vi "ReversedEngineering GetClassDependencyInfo.vi"(1 "Class/Create Path":path=path "C:/classes/P1S/EG1_class/EG1.lvclass", 5 "error in (no error)":errorcluster, 7 "Only analyse this class methods and attributes(False)":bool) -> (15 "classInfo":T5, 16 "TypeDefs":T1[](array[typedef]), 19 "error out":errorcluster)   [LabVIEW 2020]
doc: "Gets current diagram values"
uses:
  <resource>/Framework/Providers/Open_GDS/UML/ReversedEngineering/ReversedEngineering ClassInfoType.ctl
  <resource>/Framework/Providers/Open_GDS/UML/UMLEditor/UMLEditor_VisibilityType.ctl
  <resource>/Framework/Providers/Open_GDS/UML/ReversedEngineering/ReversedEngineering AttributeInfoType.ctl
  <resource>/Framework/Providers/Open_GDS/ClassProviders/Common/CommonVIs/CommonVIs_AttributeDataType.ctl
  <resource>/Framework/Providers/Open_GDS/UML/ReversedEngineering/ReversedEngineering_ClassDependencyDetailsType.ctl
  <resource>/Framework/Providers/Open_GDS/ClassProviders/Common/ScriptingFunctions/SubVIs/Scripting_ViDependencyType.ctl
  <resource>/Framework/Providers/Open_GDS/UML/ReversedEngineering/ReversedEngineering TypeDefType.ctl
  <resource>/Framework/Providers/Open_GDS/ClassProviders/Provider_BaseClassInterface/ClassReader_class/MethodDependencyType.ctl
  <resource>/Framework/Providers/Open_GDS/UML/UMLEditor/UMLEditor BusyDialogAction.ctl
  <resource>/Framework/Providers/Open_GDS/ClassProviders/Provider_BaseClassInterface/ClassReader_class/ClassReader.lvclass
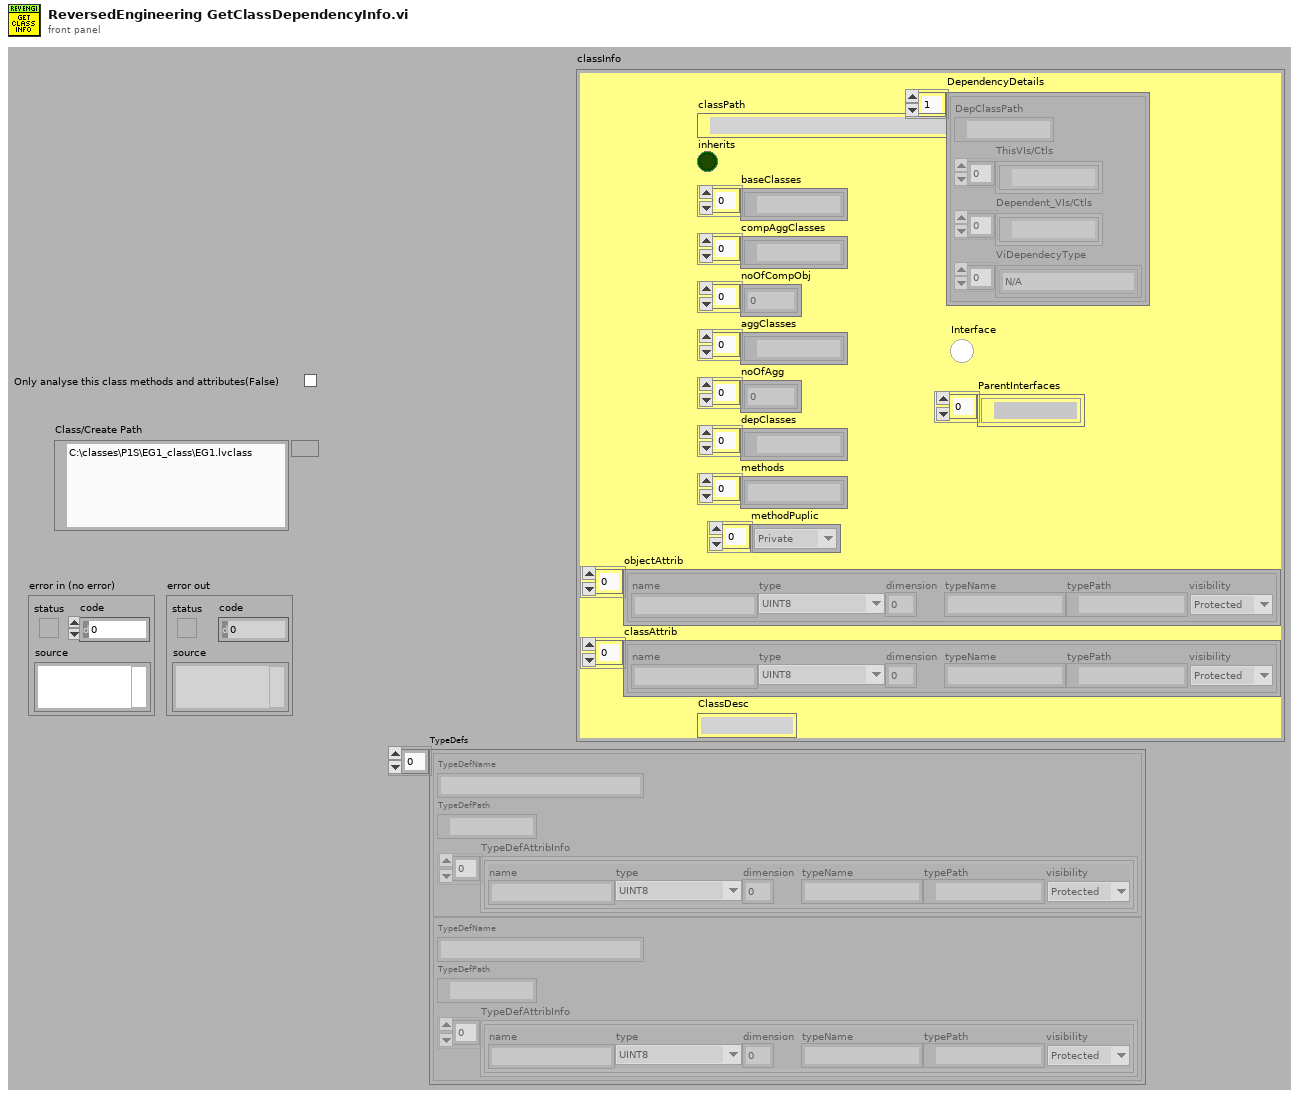
[diagram p1: front panel]
types:
  T1 = typedef "ReversedEngineering TypeDefType.ctl" = cluster{"TypeDefName":string, "TypeDefPath":path, "TypeDefAttribInfo":T2[]}
  T2 = typedef "ReversedEngineering AttributeInfoType.ctl" = cluster{"name":string, "type":T3, "dimension":i32, "typeName":string, "typePath":path, "visibility":T4}
  T3 = typedef "CommonVIs_AttributeDataType.ctl" = enum16{"UINT8", "INT8", "UINT16", "INT16", "UINT32", "INT32", "UINT64", "INT64", "SGL", "DBL", "EXT", "CSG", "CDB", "CXT", "TimeStamp", "STRING", "PATH", "BOOL", "ENUM", "RefNum", "VIRefNum", "LabVIEW Class", "Cluster", "Variant", "TypeDef", "Waveform", "LabVIEW Object", "Other", "void", "Set", "Map"}
  T4 = typedef "UMLEditor_VisibilityType.ctl" = enum16{"Public", "Private", "Protected"}
  T5 = typedef "ReversedEngineering ClassInfoType.ctl" = cluster{"classPath":path, "inherits":bool, "baseClasses":path[], "compAggClasses":path[], "noOfCompObj":i32[], "aggClasses":path[], "noOfAgg":i32[], "depClasses":path[], "methods":string[], "methodPuplic":T4[], "objectAttrib":T2[], "classAttrib":T2[], "ClassDesc":string, "DependencyDetails":T6[], "Interface":bool, "ParentInterfaces":path[]}
  T6 = typedef "ReversedEngineering_ClassDependencyDetailsType.ctl" = cluster{"DepClassPath":path, "ThisVIs/Ctls":path[], "Dependent_VIs/Ctls":path[], "ViDependecyType":T7[]}
  T7 = typedef "Scripting_ViDependencyType.ctl" = enum16{"N/A", "Launches"}
  T8 = typedef "MethodDependencyType.ctl" = cluster{"Method/VI":path, "SubVIs/Ctls":path[], "SubVIClassOwner":string[], "ClassMethodName":string[], "SubVIClassOwnerPath":path[], "DepType":T7[]}
  T9 = cluster{"inherits":bool, "baseClasses":path[], "compositeAggregationClassPath":path[], "noOfCompositeObjects":i32[], "aggregationClassPath":path[], "noOfAggObjects":i32[], "dependencyClassPath":path[], "className":string, "classPath":path, "createRef":refnum<vi>, "depClassDescRefs":refnum<vi>[], "createPath":path, "depClassNames":string[], "depClassPaths":path[], "noOfObjects1":i32[], "refData":string, "refType":i16[], "noOfObjects2":i32[], "depTypeDefsVIs":path[], "depTypeDefsClassPath":path[], "depCreateClassPaths":path[], "objectRefsInAttrib":path[], "objectRefClassesInAttrib":path[], "objectRefInAttribIsAnArray":bool[], "methodNames":string[], "objectAttribInfo":T2[], "classAttribInfo":T2[], "errMsg":string, "dirClass":bool, "CreateClassVIsCalled":path[], "TypeDefs":T1[], "ClassDesc":string, "DependencyDetails":T6[], "methodPuplic":T4[], "depMethodVIs":T8[], "DataFlowClass":bool, "IsDependencyClassPathsAByValueClass":bool[], "Interface":bool, "ParentInterfaces":path[]}
  T10 = typedef "UMLEditor BusyDialogAction.ctl" = enum16{"Initialize", "Open(VIs)", "Open(i)", "Send_I-Value", "SendStatusMessage", "GetBusyDialogStatus", "Close", "Quit"}
  T11 = enum16{"NormalSubVis", "LV-Internal VIs", "All VIs", "All Functions"}
  T12 = enum32{"invalid VI type", "Standard VI", "Control VI", "Global VI", "Polymorphic VI", "Configuration VI", "SubSystem", "Facade VI", "Method VI", "Statechart Diagram VI"}
  T13 = enum32{"invalid scope", "public", "private", "protected", "community"}
  T14 = typedef "ClassTypes_MethodType.ctl" = cluster{"MethodName":string, "Visibility":enum16{"Public", "Private", "Protected"}, "StereoType":string, "Path":path}
  T15 = typedef "Librarian File Info Out.ctl" = cluster{"creation date":u32, "last mod date":u32, "type":string, "creator":string, "LV version":i32, "size":i32, "top level":bool}
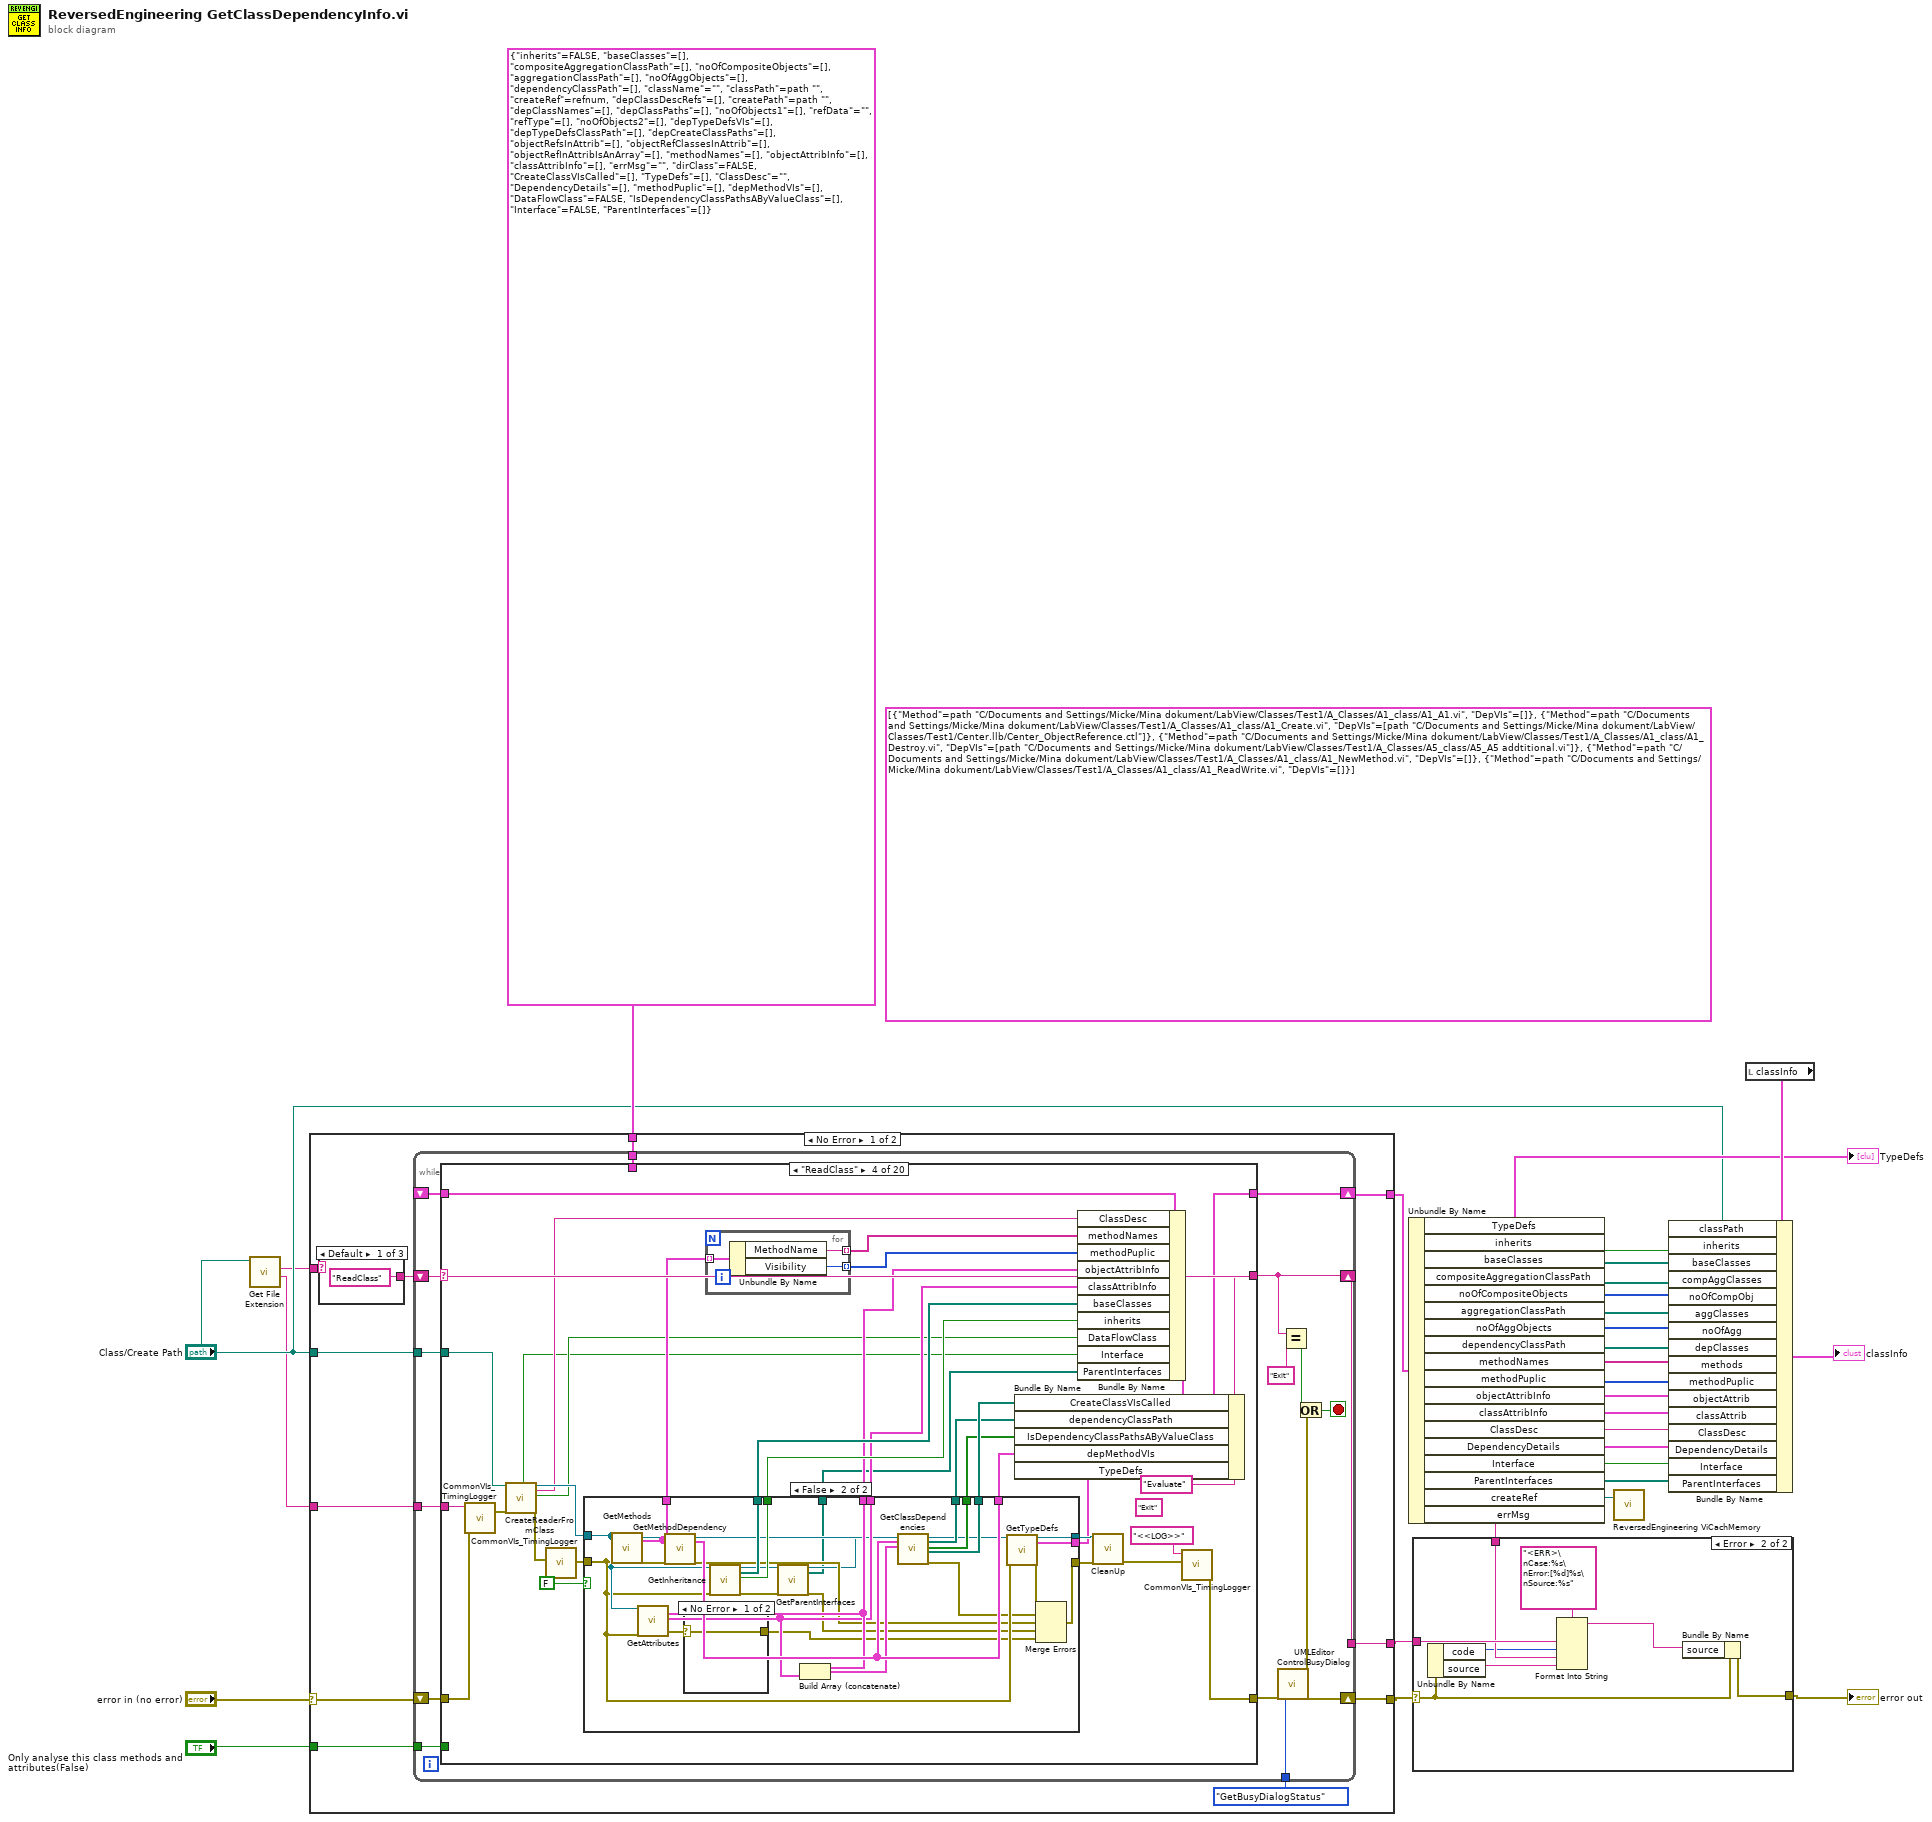
[diagram p0: block diagram]
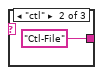
[diagram p3: hidden frame]
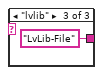
[diagram p4: hidden frame]
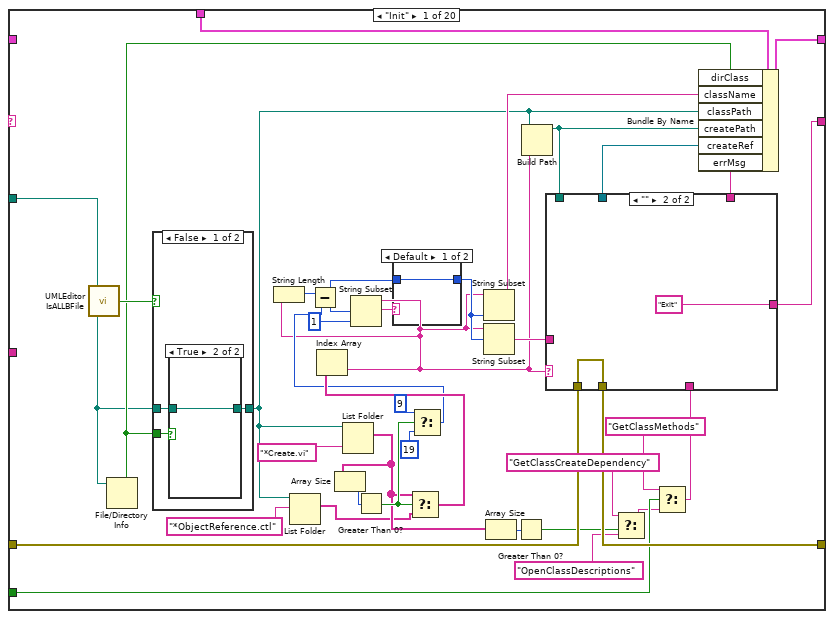
[diagram p5: hidden frame]
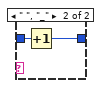
[diagram p6: hidden frame]
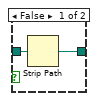
[diagram p7: hidden frame]
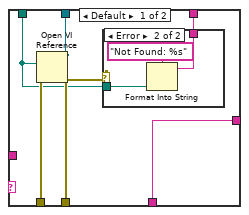
[diagram p9: hidden frame]
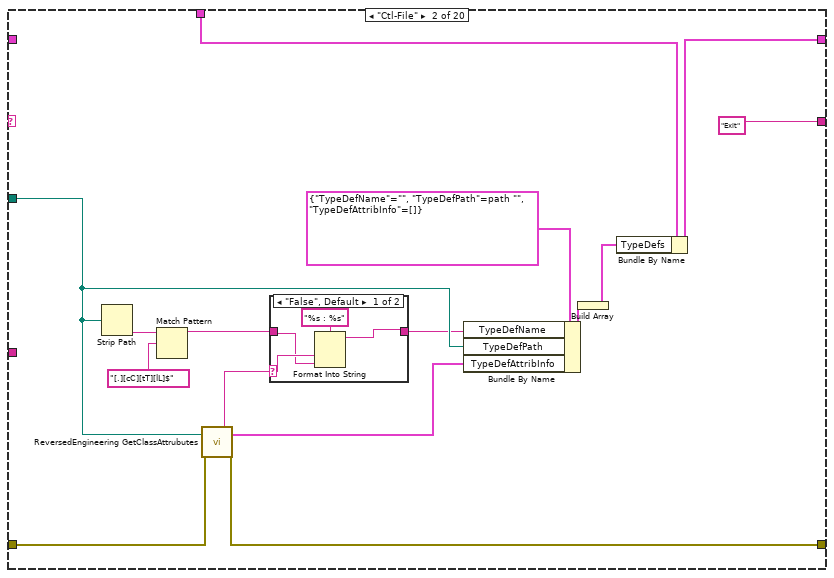
[diagram p11: hidden frame]
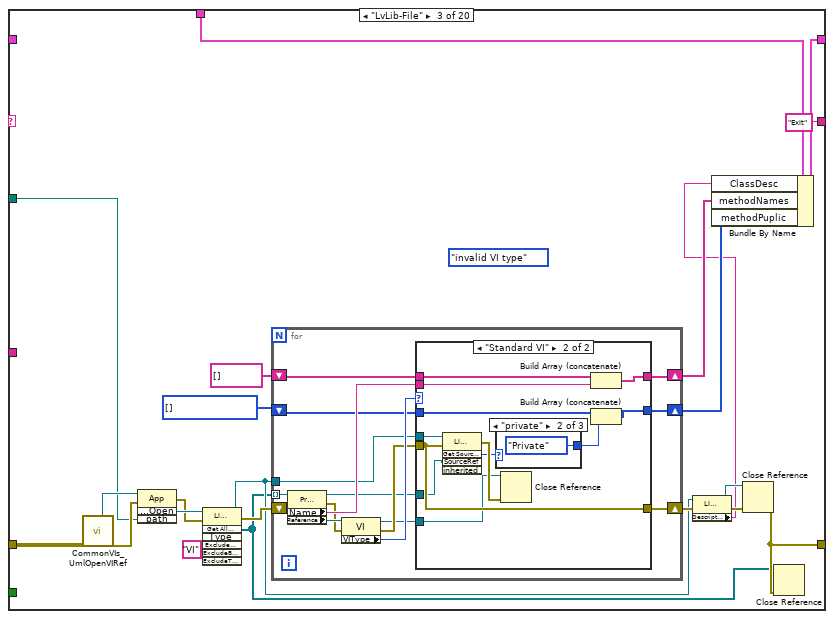
[diagram p13: hidden frame]
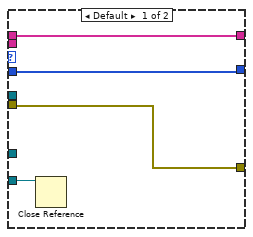
[diagram p14: hidden frame]
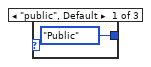
[diagram p15: hidden frame]
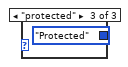
[diagram p16: hidden frame]
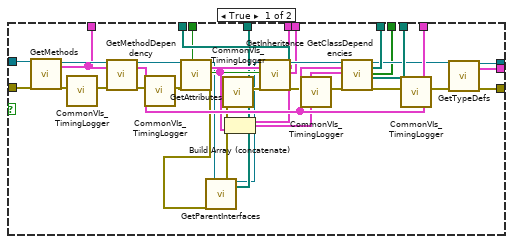
[diagram p17: hidden frame]
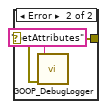
[diagram p18: hidden frame]
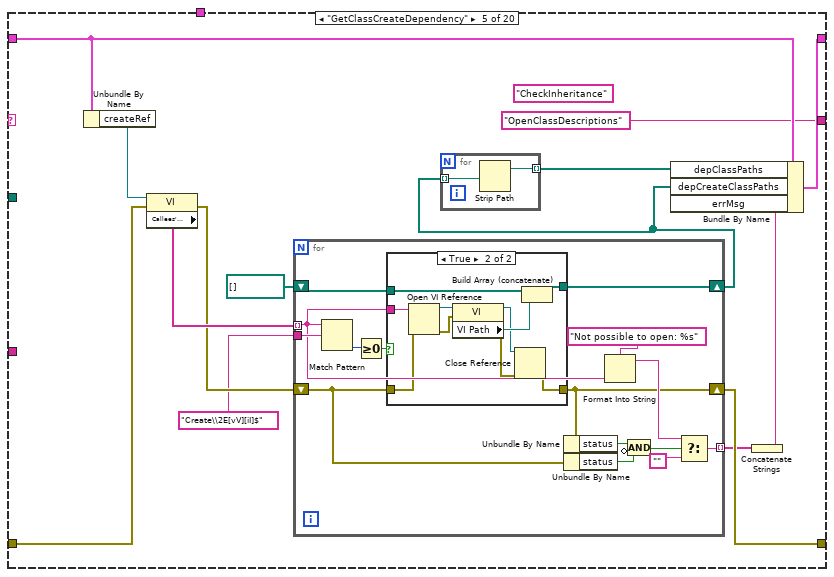
[diagram p19: hidden frame]
diagram:
  (unwired) cluster{"Method":path, "DepVIs":path[]}[] [{"Method"=path "C:/Documents and Settings/Micke/Mina dokument/LabView/Classes/Test1/A_Classes/A1_class/A1_A1.vi", "DepVIs"=[]}, {"Method"=path "C:/Documents and Settings/Micke/Mina dokument/LabView/Classes/Test1/A_Classes/A1_class/A1_Create.vi", "DepVIs"=[path "C:/Documents and Settings/Micke/Mina dokument/LabView/Classes/Test1/Center.llb/Center_ObjectReference.ctl"]}, {"Method"=path "C:/Documents and Settings/Micke/Mina dokument/LabView/Classes/Test1/A_Classes/A1_class/A1_Destroy.vi", "DepVIs"=[path "C:/Documents and Settings/Micke/Mina dokument/LabView/Classes/Test1/A_Classes/A5_class/A5_A5 addtitional.vi"]}, {"Method"=path "C:/Documents and Settings/Micke/Mina dokument/LabView/Classes/Test1/A_Classes/A1_class/A1_NewMethod.vi", "DepVIs"=[]}, {"Method"=path "C:/Documents and Settings/Micke/Mina dokument/LabView/Classes/Test1/A_Classes/A1_class/A1_ReadWrite.vi", "DepVIs"=[]}] ("depMethodVIs")
  n1 = call <vilib>:"Get File Extension.vi"("file"="Class/Create Path") -> ("filename without extension"=w3:string, "lowercase file extension"=w4:string)  [unwired: 1 in, 8 out]
  n2 = case shown="No Error" "error in (no error)" {
    selector: "error in (no error)" -> [w41 w1100]
    tunnel: [w40 w1100] -> w15
    tunnel: "Class/Create Path" -> [w39 _]
    tunnel: [w38 _] -> w29
    tunnel: [w37 _] -> w13
    tunnel: "Only analyse this class methods and attributes(False)" -> [w36 _]
    tunnel: T9 {"inherits"=FALSE, "baseClasses"=[], "compositeAggregationClassPath"=[], "noOfCompositeObjects"=[], "aggregationClassPath"=[], "noOfAggObjects"=[], "dependencyClassPath"=[], "className"="", "classPath"=path "", "createRef"=refnum, "depClassDescRefs"=[], "createPath"=path "", "depClassNames"=[], "depClassPaths"=[], "noOfObjects1"=[], "refData"="", "refType"=[], "noOfObjects2"=[], "depTypeDefsVIs"=[], "depTypeDefsClassPath"=[], "depCreateClassPaths"=[], "objectRefsInAttrib"=[], "objectRefClassesInAttrib"=[], "objectRefInAttribIsAnArray"=[], "methodNames"=[], "objectAttribInfo"=[], "classAttribInfo"=[], "errMsg"="", "dirClass"=FALSE, "CreateClassVIsCalled"=[], "TypeDefs"=[], "ClassDesc"="", "DependencyDetails"=[], "methodPuplic"=[], "depMethodVIs"=[], "DataFlowClass"=FALSE, "IsDependencyClassPathsAByValueClass"=[], "Interface"=FALSE, "ParentInterfaces"=[]} ("Cluster") -> [w34 _]
    tunnel: w4 -> [w33 _]
    tunnel: w3 -> [w31 _]
    frame No Error {
      n3 = case shown="Default" w33 {
        tunnel: ["ReadClass" ("y") "Ctl-File" "LvLib-File"] -> w32
        frame Default {
        }
        frame "ctl" {
        }
        frame "lvlib" {
        }
      }
      n4 = while {
        shift-right: [w58] -> _
        shift-left: w32 -> [w51]
        shift-right: [w45] -> w40
        shift-left: w41 -> [w59]
        shift-right: [w53] -> w38
        shift-left: _ -> [w54]
        tunnel: w39 -> [w52]
        tunnel: [w51] -> w37
        tunnel: w36 -> [w50]
        tunnel: UMLEditor_BusyDialogAction."GetBusyDialogStatus" ("Action(SendStatusMessage)") -> [w48]
        tunnel: w34 -> [w47]
        tunnel: w31 -> [w46]
        stop <- w55 stop-if-true
        n5 = case shown="\"ReadClass\"" w51 {
          tunnel: w59 -> [w87 w133 w156 w202 w306 w340 w368 w433 w479 w575 w661 w681 w703 w726 w791 w813 w879 w954 w1018 w1097]
          tunnel: [w86 w131 w140 w196 w302 w336 w369 w433 w460 w575 w666 w694 w701 w726 w791 w813 w879 w954 w1018 w1097] -> w49
          tunnel: [w96 "Exit" ("y") "Exit" ("y") "Evaluate" ("y") "OpenClassDescriptions" ("y") "CheckInheritance" ("y") "GetMultiplicity" ("y") "GetClassMethods" ("y") "GetClassMethodDepenencies" ("y") "GetObjectAttributsDepenencies" ("y") "GetClassAttributsDepenencies" ("y") "CloseRefs" ("y") "Evaluate" ("y") "RemoveInheritDependency" ("y") "CreateTypeDefs?" ("y") "AddReferencedTypeDefs" ("y") "UpdateTypeDefsAttribName?" ("y") "SortMethodToClassDependencies" ("y") "Exit" ("y") "Exit" ("y")] -> w58
          tunnel: w54 -> [_ _ _ w225 w301 w358 w365 w436 w474 w571 w668 w689 w702 w710 w789 w808 w881 w961 w1017 w1099]
          tunnel: [w95 w130 w158 w216 w300 w359 w373 w438 w475 w576 w669 w690 w702 w725 w790 w815 w880 w960 w1019 w1099] -> w53
          tunnel: w52 -> [w68 w126 w155 w226 _ _ _ _ _ _ _ _ _ _ _ _ _ _ _ _]
          tunnel: w50 -> [w71 _ _ _ _ _ _ _ _ _ _ _ _ _ _ _ _ _ _ _]
          tunnel: w47 -> [w60 w122 w141 _ _ _ _ _ _ _ _ _ _ _ _ _ _ _ _ _]
          tunnel: w46 -> [_ _ _ w201 _ _ _ _ _ _ _ _ _ _ _ _ _ _ _ _]
          frame "Init" {
            n6 = call <resource>:"UMLEditor IsALLBFile.vi"("path"=w68) -> ("path to VI library?"=w97:bool)
            n7 = File/Directory Info(path=w68) -> (directory=w84:bool)  [unwired: 1 in, 6 out]
            n8 = case shown="False" w97 {
              tunnel: w68 -> [w103 w107]
              tunnel: [w102 w107] -> w64
              tunnel: w84 -> [w101 _]
              frame False {
                n9 = case shown="True" w101 {
                  tunnel: w103 -> [w105 w106]
                  tunnel: [w104 w106] -> w102
                  frame False {
                    n10 = Strip Path(path=w105) -> (stripped path=w104:path)  [unwired: 1 out]
                  }
                  frame True {
                  }
                }
              }
              frame True {
              }
            }
            n11 = List Folder(path=w64, pattern="*ObjectReference.ctl") -> (filenames=w62:string[])  [unwired: 1 in, 4 out]
            n12 = List Folder(path=w64, pattern="*Create.vi") -> (filenames=w67:string[])  [unwired: 1 in, 4 out]
            n13 = Array Size(array=w67) -> (size(s)=w81:i32)
            n14 = Greater Than 0?(x=w81) -> (x > 0?=w79:bool)
            n15 = Select(t=w67, s=w79, f=w62) -> (s? t:f=w80:string[])
            n16 = Index Array(array=w80) -> (element=w65:string)  [unwired: 1 in]
            n17 = String Length(string=w65) -> (length=w83:i32)
            n18 = Select(t=9 ("y"), s=w79, f=19 ("y")) -> (s? t:f=w76:i32)
            n19 = Subtract(x=w83, y=w76) -> (x-y=w82:i32)
            n20 = String Subset(string=w65, offset (0)=w82, length (rest)=1 ("length (rest)")) -> (substring=w89:string)
            n21 = case shown="Default" w89 {
              tunnel: w82 -> [w98 w100]
              tunnel: [w98 w99] -> w88
              frame Default {
              }
              frame " ", "_" {
                n22 = Increment(x=w100) -> (x+1=w99:i32)
              }
            }
            n23 = String Subset(string=w65, length (rest)=w88) -> (substring=w94:string)  [unwired: 1 out]
            n24 = String Subset(string=w65, offset (0)=w88) -> (substring=w91:string)  [unwired: 1 out]
            n25 = Array Size(array=w67) -> (size(s)=w75:i32)
            n26 = Greater Than 0?(x=w75) -> (x > 0?=w74:bool)
            n27 = Build Path(base path=w64, name or relative path=w65) -> (appended path=w93:path)
            n28 = Select(t="GetClassCreateDependency", s=w74, f="OpenClassDescriptions" ("y")) -> (s? t:f=w70:string)
            n29 = Select(t="GetClassMethods" ("y"), s=w71, f=w70) -> (s? t:f=w69:string)
            n30 = case shown="\"\"" w65 {
              tunnel: [w108 "Exit"] -> w96
              tunnel: w93 -> [w110 _]
              tunnel: [w113 _] -> w92
              tunnel: w91 -> [_ _]
              tunnel: w87 -> [w112 w117]
              tunnel: [w111 w117] -> w86
              tunnel: [w109 _] -> w85
              tunnel: w69 -> [w108 _]
              frame Default {
                n31 = Open VI Reference(vi path=w110, error in (no error)=w112) -> (vi reference=w113:refnum<vi>, error out=w111:errorcluster)  [unwired: 4 out]
                n32 = case shown="Error" w111 {
                  tunnel: w110 -> [_ w115]
                  tunnel: [_ w114] -> w109
                  frame No Error {
                  }
                  frame Error {
                    n33 = Format Into String(format string="Not Found: %s", w115) -> (resulting string=w114:string)  [unwired: 2 in, 1 out]
                  }
                }
              }
              frame "" {
              }
            }
            n34 = Bundle By Name(cluster=w60, "dirClass"=w84, "className"=w94, "classPath"=w64, "createPath"=w93, "createRef"=w92, "errMsg"=w85) -> (w95:T9)
          }
          frame "Ctl-File" {
            n35 = Strip Path(path=w126) -> (name=w128:string)  [unwired: 1 out]
            n36 = Match Pattern(string=w128, regular expression="[.][cC][tT][lL]$") -> (before substring=w120:string)  [unwired: 4 out]
            n37 = call <resource>:"ReversedEngineering GetClassAttrubutes.vi"("Path(CtrlRenumf used if Path is empty)"=w126, "error in (no error)"=w133) -> ("LibraryName"=w121:string, "attributeInfo"=w125:T2[], "error out"=w131:errorcluster)  [unwired: 1 in, 14 out]
            n38 = case shown="\"False\", Default" w121 {
              selector: w121 -> [w136 _]
              tunnel: w120 -> [w134 w138]
              tunnel: [w135 w138] -> w119
              frame "False", Default {
                n39 = Format Into String(format string="%s : %s", w136, w134) -> (resulting string=w135:string)  [unwired: 2 in, 1 out]
              }
              frame "" {
              }
            }
            n40 = Bundle By Name(cluster=T1 {"TypeDefName"="", "TypeDefPath"=path "", "TypeDefAttribInfo"=[]} ("TypeDef"), "TypeDefName"=w119, "TypeDefPath"=w126, "TypeDefAttribInfo"=w125) -> (w124:T1)
            n41 = Build Array(w124) -> (w123:T1[])
            n42 = Bundle By Name(cluster=w122, "TypeDefs"=w123) -> (w130:T9)
          }
          frame "LvLib-File" {
            (unwired) T12."invalid VI type" ("VI Type")
            w149 = T4[] [] items=["Public", "Private", "Protected"]
            n43 = call <resource>:"CommonVIs_UmlOpenVIRef.vi"("error in"=w156) -> ("AppRefOut"=w157:refnum<vi>)  [unwired: 3 in, 7 out]
            n44 = invoke class="App" method="Library.Open"(reference=w157, error in=w156, "path"=w155) -> (error out=w152:errorcluster, "Open Library"=w154:refnum<vi>)  [unwired: 1 in, 2 out]
            n45 = invoke class="Library" method="Get All Descendents"(reference=w154, error in=w152, "Type"="VI") -> (reference out=w143:refnum<vi>, error out=w151:errorcluster, "All Descendents"=w139:refnum<vi>[])  [unwired: 4 in, 4 out]
            n46 = for {
              tunnel: w139 -> [w174] mode=indexing
              shift-right: [w164] -> w146
              shift-left: w151 -> [w173]
              shift-right: [w169] -> w148
              shift-left: string[] [] -> [w170]
              tunnel: w143 -> [w162]
              shift-right: [w166] -> w147
              shift-left: w149 -> [w167]
              n47 = property class="ProjectItem"(reference=w174, error in=w173) -> (reference out=w160:refnum<vi>, error out=w161:errorcluster, "Name"=w168:string, "Reference"=w172:refnum<vi>)
              n48 = property class="VI"(reference=w172, error in=w161) -> (reference out=w163:refnum<vi>, error out=w165:errorcluster, "VIType"=w171:T12)
              n49 = case shown="\"Standard VI\"" w171 {
                tunnel: w170 -> [w178 w190]
                tunnel: [w178 w187] -> w169
                tunnel: w168 -> [_ w189]
                tunnel: w167 -> [w177 w188]
                tunnel: [w177 w186] -> w166
                tunnel: w165 -> [w176 w183]
                tunnel: [w176 w183] -> w164
                tunnel: w163 -> [w175 w180]
                tunnel: w162 -> [_ w182]
                tunnel: w160 -> [_ w179]
                frame Default {
                  n50 = Close Reference(reference=w175) -> ()  [unwired: 1 in, 1 out]
                }
                frame "Standard VI" {
                  n51 = invoke class="Library" method="Get Source Scope"(reference=w182, error in=w183, "SourceRef"=w179) -> (error out=w185:errorcluster, "GetSourceScope"=w184:T13)  [unwired: 2 in, 3 out]
                  n52 = case shown="\"private\"" w184 {
                    tunnel: [UMLEditor_VisibilityType."Public" ("Enum") UMLEditor_VisibilityType."Private" ("Enum") UMLEditor_VisibilityType."Protected" ("Enum")] -> w181
                    frame "public", Default {
                    }
                    frame "private" {
                    }
                    frame "protected" {
                    }
                  }
                  n53 = Close Reference(reference=w180, error in (no error)=w185) -> ()  [unwired: 1 out]
                  n54 = Build Array (concatenate)(w190, w189) -> (w187:string[])
                  n55 = Build Array (concatenate)(w188, w181) -> (w186:T4[])
                }
              }
            }
            n56 = property class="Library"(reference=w143, error in=w146) -> (reference out=w144:refnum<vi>, error out=w145:errorcluster, "Description"=w142:string)
            n57 = Bundle By Name(cluster=w141, "ClassDesc"=w142, "methodNames"=w148, "methodPuplic"=w147) -> (w158:T9)
            n58 = Close Reference(reference=w144, error in (no error)=w145) -> (error out=w140:errorcluster)
            n59 = Close Reference(reference=w139, error in (no error)=w140) -> ()  [unwired: 1 out]
          }
          frame "ReadClass" {
            (unwired) "Exit" ("y")
            n60 = call <resource>:"CommonVIs_TimingLogger.vi"("error in (no error)"=w202, "Name"=w201) -> ("error out"=w203:errorcluster)  [unwired: 9 in]
            n61 = call <resource>:"CreateReaderFromClass.vi"("ClassPath/LvClassRef"=w226, "error in"=w203) -> ("Is Interface"=w195:bool, "ClassReader"=w224:refnum<class "ClassReader.lvclass">, "Description"=w223:string, "DataFlowClass"=w209:bool, "error out"=w200:errorcluster)  [unwired: 13 out]
            n62 = call <resource>:"CommonVIs_TimingLogger.vi"("error in (no error)"=w200) -> ("error out"=w199:errorcluster)  [unwired: 10 in]
            n63 = case shown="False" FALSE {
              tunnel: w199 -> [w259 w273]
              tunnel: w224 -> [w258 w275]
              tunnel: [w257 w286] -> w220
              tunnel: [w256 w285] -> w219
              tunnel: [w254 w284] -> w218
              tunnel: [w251 w283] -> w215
              tunnel: [w250 w282] -> w214
              tunnel: [w249 w281] -> w213
              tunnel: [w248 w280] -> w211
              tunnel: [w247 w279] -> w210
              tunnel: [w244 w278] -> w208
              tunnel: [w243 w274] -> w207
              tunnel: [w242 w277] -> w206
              tunnel: [w241 w276] -> w205
              tunnel: [w229 w260] -> w194
              frame True {
                n64 = call-dynamic "GetMethods.vi"("ClassReader in"=w258, "error in (no error)"=w259) -> ("ClassReader out"=w255:refnum<class "ClassReader.lvclass">, "Methods"=w254:T14[], "error out"=w240:errorcluster)  [unwired: 15 out]
                n65 = call <resource>:"CommonVIs_TimingLogger.vi"("error in (no error)"=w240) -> ("error out"=w239:errorcluster)  [unwired: 10 in]
                n66 = call-dynamic "GetMethodDependency.vi"("ClassReader in"=w255, "Method(s)"=w254, "error in (no error)"=w239) -> ("ClassReader out"=w253:refnum<class "ClassReader.lvclass">, "DependencyVIs"=w249:T8[], "error out"=w238:errorcluster)  [unwired: 14 out]
                n67 = call <resource>:"CommonVIs_TimingLogger.vi"("error in (no error)"=w238) -> ("error out"=w237:errorcluster)  [unwired: 10 in]
                n68 = call-dynamic "GetAttributes.vi"("ClassReader in"=w253, "error in (no error)"=w237) -> ("ClassReader out"=w228:refnum<class "ClassReader.lvclass">, "ObjectAttributes"=w248:T2[], "ClassAttributes"=w247:T2[], "error out"=w231:errorcluster)  [unwired: 1 in, 13 out]
                n69 = call-dynamic "GetParentInterfaces.vi"("ClassReader in"=w228, "error in (no error)"=w231) -> ("ClassReader out"=w227:refnum<class "ClassReader.lvclass">, "ParentInterfaces"=w229:path[], "error out"=w230:errorcluster)  [unwired: 15 in]
                n70 = call <resource>:"CommonVIs_TimingLogger.vi"("error in (no error)"=w230) -> ("error out"=w236:errorcluster)  [unwired: 10 in]
                n71 = Build Array (concatenate)(w248, w247) -> (w246:T2[])
                n72 = call-dynamic "GetInheritance.vi"("ClassReader in"=w227, "error in (no error)"=w236) -> ("ClassReader out"=w252:refnum<class "ClassReader.lvclass">, "Inheritance"=w257:path[], "Inherits"=w256:bool, "error out"=w234:errorcluster)  [unwired: 14 out]
                n73 = call <resource>:"CommonVIs_TimingLogger.vi"("error in (no error)"=w234) -> ("error out"=w235:errorcluster)  [unwired: 10 in]
                n74 = call-dynamic "GetClassDependencies.vi"("ClassReader in"=w252, "DependencyVIs"=w249, "Attributes"=w246, "error in (no error)"=w235) -> ("ClassReader out"=w245:refnum<class "ClassReader.lvclass">, "DependencyClassPaths"=w250:path[], "IsDependencyClassPathsAByValueClass"=w241:bool[], "CreateClassVIsCalled"=w251:path[], "error out"=w233:errorcluster)  [unwired: 11 out]
                n75 = call <resource>:"CommonVIs_TimingLogger.vi"("error in (no error)"=w233) -> ("error out"=w232:errorcluster)  [unwired: 10 in]
                n76 = call-dynamic "GetTypeDefs.vi"("ClassReader in"=w245, "error in (no error)"=w232) -> ("ClassReader out"=w244:refnum<class "ClassReader.lvclass">, "TypeDefs"=w242:T1[], "error out"=w243:errorcluster)  [unwired: 15 out]
              }
              frame False {
                n77 = call-dynamic "GetMethods.vi"("ClassReader in"=w275, "error in (no error)"=w273) -> ("ClassReader out"=w272:refnum<class "ClassReader.lvclass">, "Methods"=w284:T14[], "error out"=w271:errorcluster)  [unwired: 15 out]
                n78 = call-dynamic "GetAttributes.vi"("ClassReader in"=w275, "error in (no error)"=w273) -> ("ObjectAttributes"=w280:T2[], "ClassAttributes"=w279:T2[], "error out"=w268:errorcluster)  [unwired: 1 in, 14 out]
                n79 = call-dynamic "GetMethodDependency.vi"("ClassReader in"=w272, "Method(s)"=w284, "error in (no error)"=w271) -> ("DependencyVIs"=w281:T8[], "error out"=w266:errorcluster)  [unwired: 15 out]
                n80 = case shown="No Error" w268 {
                  selector: w268 -> [w287 w289]
                  tunnel: [w287 w289] -> w265
                  frame No Error {
                  }
                  frame Error {
                    n81 = call <resource>:"GOOP_DebugLogger.vi"("error in (no error)"=w289, "State"="GetAttributes") -> ()  [unwired: 7 in, 3 out]
                  }
                }
                n82 = call-dynamic "GetInheritance.vi"("ClassReader in"=w275, "error in (no error)"=w273) -> ("ClassReader out"=w263:refnum<class "ClassReader.lvclass">, "Inheritance"=w286:path[], "Inherits"=w285:bool, "error out"=w264:errorcluster)  [unwired: 14 out]
                n83 = call-dynamic "GetParentInterfaces.vi"("ClassReader in"=w263, "error in (no error)"=w264) -> ("ClassReader out"=w262:refnum<class "ClassReader.lvclass">, "ParentInterfaces"=w260:path[], "error out"=w261:errorcluster)  [unwired: 15 in]
                n84 = Build Array (concatenate)(w280, w279) -> (w269:T2[])
                n85 = call-dynamic "GetClassDependencies.vi"("ClassReader in"=w262, "DependencyVIs"=w281, "Attributes"=w269) -> ("DependencyClassPaths"=w282:path[], "IsDependencyClassPathsAByValueClass"=w276:bool[], "CreateClassVIsCalled"=w283:path[], "error out"=w267:errorcluster)  [unwired: 1 in, 12 out]
                n86 = call-dynamic "GetTypeDefs.vi"("ClassReader in"=w275, "error in (no error)"=w273) -> ("ClassReader out"=w278:refnum<class "ClassReader.lvclass">, "TypeDefs"=w277:T1[], "error out"=w270:errorcluster)  [unwired: 15 out]
                n87 = Merge Errors(w270, w267, w266, w261, w265) -> (w274:errorcluster)
              }
            }
            n88 = for {
              tunnel: w218 -> [w292] mode=indexing
              tunnel: [w291] -> w222 mode=indexing
              tunnel: [w290] -> w221 mode=indexing
              n89 = Unbundle By Name(w292) -> ("MethodName"=w291:string, "Visibility"=w290:enum16{"Public", "Private", "Protected"})
            }
            n90 = Bundle By Name(cluster=w225, "ClassDesc"=w223, "methodNames"=w222, "methodPuplic"=w221, "objectAttribInfo"=w211, "classAttribInfo"=w210, "baseClasses"=w220, "inherits"=w219, "DataFlowClass"=w209, "Interface"=w195, "ParentInterfaces"=w194) -> (w217:T9)
            n91 = Bundle By Name(cluster=w217, "CreateClassVIsCalled"=w215, "dependencyClassPath"=w214, "IsDependencyClassPathsAByValueClass"=w205, "depMethodVIs"=w213, "TypeDefs"=w206) -> (w216:T9)
            n92 = call-dynamic "CleanUp.vi"("reference in"=w208, "error in (no error)"=w207) -> ("error out"=w197:errorcluster)  [unwired: 17 out]
            n93 = call <resource>:"CommonVIs_TimingLogger.vi"("error in (no error)"=w197, "Name"="<<LOG>>") -> ("error out"=w196:errorcluster)  [unwired: 9 in]
          }
          frame "GetClassCreateDependency" {
            (unwired) "CheckInheritance" ("y")
            n94 = Unbundle By Name(w301) -> ("createRef"=w294:refnum<vi>)
            n95 = property class="VI"(reference=w294, error in=w306) -> (error out=w304:errorcluster, "Callees' Names"=w305:string[])  [unwired: 1 out]
            n96 = for {
              tunnel: w305 -> [w309] mode=indexing
              shift-right: [w320] -> w296
              shift-left: path[] [] -> [w321]
              shift-right: [w312] -> w302
              shift-left: w304 -> [w311]
              tunnel: "Create\\2E[vV][iI]$" ("regular expression") -> [w319]
              tunnel: [w310] -> w297 mode=indexing
              n97 = Match Pattern(string=w309, regular expression=w319) -> (offset past match=w323:i32)  [unwired: 4 out]
              n98 = Greater Or Equal To 0?(x=w323) -> (x >= 0?=w322:bool)
              n99 = case shown="True" w322 {
                tunnel: w321 -> [w325 w335]
                tunnel: w309 -> [_ w334]
                tunnel: w311 -> [w324 w333]
                tunnel: [w325 w329] -> w320
                tunnel: [w324 w326] -> w312
                frame False {
                }
                frame True {
                  n100 = Open VI Reference(vi path=w334, error in (no error)=w333) -> (vi reference=w332:refnum<vi>, error out=w331:errorcluster)  [unwired: 1 in, 3 out]
                  n101 = property class="VI"(reference=w332, error in=w331) -> (reference out=w327:refnum<vi>, error out=w328:errorcluster, "VI Path"=w330:path)
                  n102 = Close Reference(reference=w327, error in (no error)=w328) -> (error out=w326:errorcluster)
                  n103 = Build Array (concatenate)(w335, w330) -> (w329:path[])
                }
              }
              n104 = Unbundle By Name(w312) -> ("status"=w318:bool)
              n105 = Unbundle By Name(w311) -> ("status"=w317:bool)
              n106 = Format Into String(format string="Not possible to open: %s", w309) -> (resulting string=w313:string)  [unwired: 2 in, 1 out]
              n107 = Compound Arithmetic op=AND(w318, invert w317) -> (w316:bool)
              n108 = Select(t=w313, s=w316, f="") -> (s? t:f=w310:string)
            }
            n109 = for {
              tunnel: w296 -> [w308] mode=indexing
              tunnel: [w307] -> w299 mode=indexing
              n110 = Strip Path(path=w308) -> (stripped path=w307:path)  [unwired: 1 out]
            }
            n111 = Concatenate Strings(w297) -> (w295:string)
            n112 = Bundle By Name(cluster=w301, "depClassPaths"=w299, "depCreateClassPaths"=w296, "errMsg"=w295) -> (w300:T9)
          }
          frame "OpenClassDescriptions" {
            n113 = Unbundle By Name(w358) -> ("classPath"=w344:path)
            n114 = call <resource>:"CommonVIs_ListFilesRecursive.vi"("directory path"=w344, "FileSearchPattern"="*ClassDescription.vi", "error in (no error)"=w340) -> ("Files"=w342:path[], "error out"=w339:errorcluster)  [unwired: 3 in, 12 out]
            n115 = Index Array(array=w342) -> (element=w341:path)  [unwired: 1 in]
            n116 = Open VI Reference(vi path=w341, error in (no error)=w339) -> (vi reference=w350:refnum<vi>, error out=w351:errorcluster)  [unwired: 1 in, 3 out]
            n117 = Unbundle By Name(w351) -> ("status"=w357:bool)
            n118 = Unbundle By Name(w339) -> ("status"=w356:bool)
            n119 = invoke class="VI" method="Ctrl Val.Get"(reference=w350, error in=w351, "Control Name"="Class description") -> (reference out=w337:refnum<vi>, error out=w338:errorcluster, "Get Control Value Variant"=w347:variant)  [unwired: 1 in, 1 out]
            n120 = Format Into String(format string="Not Found: %s", w341) -> (resulting string=w352:string)  [unwired: 2 in, 1 out]
            n121 = Compound Arithmetic op=AND(w357, invert w356) -> (w355:bool)
            n122 = Select(t=w352, s=w355, f="") -> (s? t:f=w346:string)
            n123 = Variant To Data(type=w346, Variant=w347) -> (data=w345:string)  [unwired: 1 in, 1 out]
            n124 = call <resource>:"ReversedEngineering ViCachMemory.vi"("ViRef"=w337, "error in (no error)"=w338) -> ("error out"=w336:errorcluster)  [unwired: 2 in, 15 out]
            n125 = Bundle By Name(cluster=w358, "errMsg"=w346, "ClassDesc"=w345) -> (w359:T9)
          }
          frame "CheckInheritance" {
            n126 = Unbundle By Name(w365) -> ("dirClass"=w364:bool)  [unwired: 1 out]
            n127 = Unbundle By Name(w365) -> ("classPath"=w363:path, "className"=w376:string)
            n128 = Concatenate Strings(w376, "GOOPKernel.vi" ("string")) -> (w374:string)
            n129 = case shown="True" w364 {
              tunnel: w363 -> [w377 w380]
              tunnel: [w377 w379] -> w362
              tunnel: "private" ("element") -> [_ w378]
              frame False {
              }
              frame True {
                n130 = Build Path(base path=w380, name or relative path=w378) -> (appended path=w379:path)
              }
            }
            n131 = Build Path(base path=w362, name or relative path=w374) -> (appended path=w367:path)
            n132 = while {
              tunnel: [w387] -> w372 mode=indexing
              shift-right: [w386] -> w369
              shift-left: w368 -> [w388]
              tunnel: [w385] -> w360 mode=indexing
              shift-right: [w383] -> _
              shift-left: w367 -> [w384]
              shift-right: [w381] -> w366
              shift-left: w365 -> [w382]
              stop <- w387 continue-if-true
              n133 = Open VI Reference(vi path=w384, error in (no error)=w388) -> (vi reference=w395:refnum<vi>, error out=w394:errorcluster)  [unwired: 4 out]
              n134 = property class="VI"(reference=w395, error in=w394) -> (reference out=w385:refnum<vi>, error out=w389:errorcluster, "Callees' Names"=w393:string[])
              n135 = Array Size(array=w393) -> (size(s)=w391:i32)
              n136 = while {
                tunnel: w393 -> [w419] mode=indexing
                tunnel: "GOOPKernel.[vV][iI]$" ("string") -> [w426]
                tunnel: w391 -> [w417]
                tunnel: [w421] -> w387
                tunnel: [w420] -> _
                tunnel: [w419] -> w390
                i -> [w425]
                stop <- w422 stop-if-true
                n137 = Increment(x=w425) -> (x+1=w418:i32)
                n138 = Match Pattern(string=w419, regular expression=w426) -> (before substring=w420:string, offset past match=w424:i32)  [unwired: 3 out]
                n139 = Greater Or Equal?(x=w418, y=w417) -> (x >= y?=w423:bool)
                n140 = Greater Or Equal To 0?(x=w424) -> (x >= 0?=w421:bool)
                n141 = Or(x=w421, y=w423) -> (x .or. y?=w422:bool)
              }
              n142 = case shown="True" w387 {
                tunnel: w390 -> [_ w413]
                tunnel: w389 -> [w398 w408]
                tunnel: [w398 w407] -> w386
                tunnel: w382 -> [w397 w405]
                tunnel: [w397 w406] -> w381
                tunnel: [path "" ("Path") w402] -> w383
                frame False {
                }
                frame True {
                  # "Iheritance"
                  n143 = Unbundle By Name(w405) -> ("baseClasses"=w404:path[])
                  n144 = Open VI Reference(vi path=w413, error in (no error)=w408) -> (vi reference=w412:refnum<vi>, error out=w411:errorcluster)  [unwired: 4 out]
                  n145 = property class="VI"(reference=w412, error in=w411) -> (reference out=w410:refnum<vi>, error out=w409:errorcluster, "VI Path"=w402:path)
                  n146 = Strip Path(path=w402) -> (stripped path=w400:path)  [unwired: 1 out]
                  n147 = call <resource>:"UMLEditor IsALLBFile.vi"("path"=w400) -> ("path to VI library?"=w401:bool)
                  n148 = case shown="False" w401 {
                    tunnel: [w414 w416] -> w399
                    tunnel: w400 -> [w415 w416]
                    frame False {
                      n149 = Strip Path(path=w415) -> (stripped path=w414:path)  [unwired: 1 out]
                    }
                    frame True {
                    }
                  }
                  n150 = Build Array (concatenate)(w404, w399) -> (w403:path[])
                  n151 = Bundle By Name(cluster=w405, "baseClasses"=w403) -> (w406:T9)
                  n152 = Close Reference(reference=w410, error in (no error)=w409) -> (error out=w407:errorcluster)
                }
              }
            }
            n153 = Or Array Elements(Boolean array=w372) -> (logical OR=w370:bool)
            n154 = Bundle By Name(cluster=w366, "inherits"=w370) -> (w373:T9)
            n155 = call <resource>:"ReversedEngineering ViCachMemory.vi"("ViRef-Array"=w360) -> ()  [unwired: 3 in, 16 out]
          }
          frame "GetMultiplicity" {
            n156 = Unbundle By Name(w436) -> ("depCreateClassPaths"=w441:path[], "createRef"=w442:refnum<vi>)
            n157 = Unbundle By Name(w436) -> ("baseClasses"=w435:path[])
            n158 = property class="VI"(reference=w442) -> ("Block Diagram"=w432:refnum<vi>)  [unwired: 1 in, 2 out]
            n159 = Index Array(array=w435) -> (element=w434:path)  [unwired: 1 in]
            n160 = call <resource>:"ReversedEngineering GetDiagramSubVIs.vi"("Diagram"=w432, "SubVIsOptions(NormalSubVis)"=T11."NormalSubVis", "RecrsiveSearchInNormalSubVIs(False)"=FALSE, "error in (no error)"=errorcluster {"status"=FALSE, "code"=0, "source"=""}, "PathToDebugVI(OnlyUsedForRecursivVitFiles)"=path "") -> ("DiagramOut"=w431:refnum<vi>, "SubViNames"=w440:string[])  [unwired: 13 out]
            n161 = Close Reference(reference=w431) -> ()  [unwired: 1 in, 1 out]
            n162 = for {
              tunnel: w441 -> [w444] mode=indexing
              tunnel: w440 -> [w451]
              tunnel: [w447] -> w439 mode=indexing
              tunnel: w434 -> [w446]
              n163 = Strip Path(path=w444) -> (stripped path=w443:path, name=w450:string)
              n164 = Equal?(x=w446, y=w443) -> (x = y?=w445:bool)
              n165 = for {
                tunnel: w451 -> [w458] mode=indexing
                tunnel: w450 -> [w457]
                tunnel: [w455] -> w449 mode=indexing
                n166 = Equal?(x=w457, y=w458) -> (x = y?=w456:bool)
                n167 = Boolean To (0,1)(Boolean=w456) -> (0, 1=w455:i16)
              }
              n168 = Add Array Elements(numeric array=w449) -> (sum=w448:i16)
              n169 = case shown="True" w445 {
                tunnel: w448 -> [w452 w454]
                tunnel: [w452 w453] -> w447
                frame False {
                }
                frame True {
                  n170 = Decrement(x=w454) -> (x-1=w453:i16)
                }
              }
            }
            n171 = Bundle By Name(cluster=w436, "noOfObjects1"=w439) -> (w438:T9)
          }
          frame "GetClassMethods" {
            w459 = T8[] []  # depMethodVIs
            n172 = Unbundle By Name(w474) -> ("className"=w466:string, "classPath"=w463:path)
            n173 = Unbundle By Name(w474) -> ("dirClass"=w468:bool, "classPath"=w467:path)
            n174 = List Folder(path=w463, pattern="*.vi", error in=w479) -> (path out=w482:path, filenames=w481:string[], error out=w476:errorcluster)  [unwired: 2 out]
            n175 = for {
              tunnel: w482 -> [w564]
              tunnel: w481 -> [w562] mode=indexing
              tunnel: [w563] -> w480 mode=indexing
              n176 = Build Path(base path=w564, name or relative path=w562) -> (appended path=w563:path)
            }
            n177 = case shown="False" w468 {
              tunnel: w467 -> [_ w489]
              tunnel: [path[] [] w486] -> w465
              frame False {
              }
              frame True {
                n178 = List Folder(path=w489) -> (path out=w488:path, folder names=w487:string[])  [unwired: 1 in, 4 out]
                n179 = for {
                  tunnel: w488 -> [w493]
                  tunnel: w487 -> [w490] mode=indexing
                  shift-right: [w491] -> w486
                  shift-left: path[] [] -> [w492]
                  n180 = case shown="Default" w490 {
                    tunnel: w493 -> [_ w500]
                    tunnel: w490 -> [_ w499]
                    tunnel: w492 -> [w494 w497]
                    tunnel: [w494 w496] -> w491
                    frame "Example", "Examples", "Test" {
                    }
                    frame Default {
                      n181 = Build Path(base path=w500, name or relative path=w499) -> (appended path=w498:path)
                      n182 = List Folder(path=w498, pattern="*.vi") -> (path out=w502:path, filenames=w503:string[])  [unwired: 1 in, 3 out]
                      n183 = for {
                        tunnel: w502 -> [w506]
                        tunnel: w503 -> [w504] mode=indexing
                        tunnel: [w505] -> w495 mode=indexing
                        n184 = Build Path(base path=w506, name or relative path=w504) -> (appended path=w505:path)
                      }
                      n185 = Build Array (concatenate)(w497, w495) -> (w496:path[])
                    }
                  }
                }
              }
            }
            n186 = Build Array (concatenate)(w480, w465) -> (w464:path[])
            n187 = call <resource>:"ReversedEngineering HideClassMethods.vi"("Item Paths"=w464, "error in (no error)"=w476) -> ("Item Paths filtered"=w478:path[], "error out"=w477:errorcluster)  [unwired: 16 out]
            n188 = for {
              tunnel: w478 -> [w513] mode=indexing
              shift-right: [w518] -> w461
              shift-left: w477 -> [w534]
              shift-right: [w516] -> w473
              shift-left: w459 -> [w515]
              tunnel: [w510] -> w471 mode=indexing
              tunnel: "[.][vV][iI][tT]*$" ("regular expression") -> [w530]
              tunnel: [w529] -> w469 mode=indexing
              tunnel: w466 -> [w524]
              tunnel: w463 -> [w520]
              tunnel: [w519] -> w462 mode=indexing
              n189 = Strip Path(path=w513) -> (stripped path=w527:path, name=w525:string)
              n190 = call <resource>:"UMLEditor IsALLBFile.vi"("path"=w527) -> ("path to VI library?"=w528:bool)
              n191 = case shown="False" w528 {
                tunnel: [w537 w541] -> w511
                tunnel: w513 -> [_ w540]
                tunnel: w527 -> [w539 _]
                tunnel: w520 -> [w538 _]
                frame False {
                  n192 = Equal?(x=w539, y=w538) -> (x = y?=w537:bool)
                }
                frame True {
                  n193 = call <vilib>:"Get VI Library File Info.vi"("path"=w540) -> ("file information"=w542:T15)  [unwired: 1 in, 9 out]
                  n194 = Unbundle By Name(w542) -> ("top level"=w541:bool)
                }
              }
              n195 = Open VI Reference(vi path=w513, error in (no error)=w534) -> (vi reference=w536:refnum<vi>, error out=w535:errorcluster)  [unwired: 4 out]
              n196 = Match Pattern(string=w525, regular expression=w524) -> (before substring=w523:string, after substring=w522:string, offset past match=w526:i32)  [unwired: 2 out]
              n197 = property class="VI"(reference=w536, error in=w535) -> (reference out=w519:refnum<vi>, error out=w532:errorcluster, "Callees' Names"=w533:string[])
              n198 = Concatenate Strings(w523, w522) -> (w521:string)
              n199 = Match Pattern(string=w521, regular expression=w530, offset (0)=w526) -> (before substring=w529:string)  [unwired: 3 out]
              n200 = Select(t=UMLEditor_VisibilityType."Public" ("Enum"), s=w511, f=UMLEditor_VisibilityType."Private" ("Enum")) -> (s? t:f=w510:T4)
              n201 = for {
                tunnel: w533 -> [w543] mode=indexing
                shift-right: [w548] -> w518
                shift-left: w532 -> [w549]
                tunnel: "[.][~.]+$" ("regular expression") -> [w547]
                shift-right: [w544] -> w514
                shift-left: path[] [] -> [w545]
                n202 = Match Pattern(string=w543, regular expression=w547) -> (offset past match=w546:i32)  [unwired: 4 out]
                n203 = case shown="0.." w546 {
                  tunnel: w549 -> [w551 w561]
                  tunnel: [w551 w556] -> w548
                  tunnel: w543 -> [_ w555]
                  tunnel: w545 -> [w550 w553]
                  tunnel: [w550 w554] -> w544
                  frame Default {
                  }
                  frame 0.. {
                    n204 = Open VI Reference(vi path=w555, error in (no error)=w561) -> (vi reference=w558:refnum<vi>, error out=w557:errorcluster)  [unwired: 4 out]
                    n205 = property class="VI"(reference=w558, error in=w557) -> (reference out=w560:refnum<vi>, error out=w559:errorcluster, "VI Path"=w552:path)
                    n206 = Build Array (concatenate)(w553, w552) -> (w554:path[])
                    n207 = Close Reference(reference=w560, error in (no error)=w559) -> (error out=w556:errorcluster)
                  }
                }
              }
              n208 = Bundle(cluster=T8 {"Method/VI"=path "", "SubVIs/Ctls"=[], "SubVIClassOwner"=[], "ClassMethodName"=[], "SubVIClassOwnerPath"=[], "DepType"=[]}, "Method/VI"=w513, "SubVIs/Ctls"=w514) -> (w512:T8)  [unwired: 4 out]
              n209 = Build Array (concatenate)(w515, w512) -> (w516:T8[])
            }
            n210 = Bundle By Name(cluster=w474, "methodNames"=w469, "methodPuplic"=w471, "depMethodVIs"=w473) -> (w475:T9)
            n211 = call <resource>:"ReversedEngineering ViCachMemory.vi"("ViRef-Array"=w462, "error in (no error)"=w461) -> ("error out"=w460:errorcluster)  [unwired: 2 in, 15 out]
          }
          frame "GetClassMethodDepenencies" {
            w566 = path[] []
            n212 = Unbundle By Name(w571) -> ("dirClass"=w573:bool, "classPath"=w572:path, "depMethodVIs"=w569:T8[])
            n213 = Unbundle By Name(w571) -> ("baseClasses"=w570:path[])
            n214 = for {
              tunnel: w573 -> [w589]
              tunnel: w572 -> [w588]
              tunnel: w570 -> [w587]
              tunnel: w569 -> [w577] mode=indexing
              shift-right: [w585] -> w568
              shift-left: w566 -> [w586]
              shift-right: [w584] -> w567
              shift-left: w566 -> [w583]
              tunnel: w566 -> [w581]
              tunnel: [w578] -> w565 mode=indexing
              n215 = Unbundle(w577) -> ("Method/VI"=w579:path, "SubVIs/Ctls"=w582:path[])  [unwired: 4 out]
              n216 = for {
                shift-right: [w628] -> w585
                shift-left: w586 -> [w629]
                tunnel: w589 -> [w622]
                tunnel: w588 -> [w621]
                shift-right: [w611] -> w584
                shift-left: w583 -> [w612]
                tunnel: w587 -> [w606]
                tunnel: w582 -> [w594] mode=indexing
                shift-right: [w593] -> w580
                shift-left: w581 -> [w595]
                w619 = "*GOOPKernel.vi" ("pattern")
                # "Its a Class Method"
                n217 = Strip Path(path=w594) -> (stripped path=w600:path, name=w610:string)
                n218 = Match Pattern(string=w610, regular expression="[Cc][Rr][Ee][Aa][Tt][Ee].vi$" ("string")) -> (offset past match=w608:i32)  [unwired: 4 out]
                n219 = for {
                  tunnel: w610 -> [w652]
                  tunnel: string[] ["ObjectAttributes.ctl$", "ClassAttributes.ctl$"] -> [w651] mode=indexing
                  tunnel: [w649] -> w624 mode=indexing
                  n220 = Match Pattern(string=w652, regular expression=w651) -> (offset past match=w650:i32)  [unwired: 4 out]
                  n221 = Greater Or Equal To 0?(x=w650) -> (x >= 0?=w649:bool)
                }
                n222 = List Folder(path=w600, pattern=w619) -> (filenames=w627:string[])  [unwired: 1 in, 4 out]
                n223 = Greater Or Equal To 0?(x=w608) -> (x >= 0?=w607:bool)
                n224 = Build Path(base path=w600, name or relative path="private" ("element")) -> (appended path=w620:path)
                n225 = Search 1D Array(1D array=w606, element=w600) -> (index of element=w605:i32)  [unwired: 1 out]
                n226 = List Folder(path=w620, pattern=w619) -> (filenames=w618:string[])  [unwired: 1 in, 4 out]
                n227 = Or Array Elements(Boolean array=w624) -> (logical OR=w623:bool)
                n228 = Array Size(array=w627) -> (size(s)=w626:i32)
                n229 = case shown="False" w622 {
                  tunnel: [w641 w646] -> w596
                  tunnel: w600 -> [w640 w648]
                  tunnel: w621 -> [w639 w642]
                  frame False {
                    n230 = Not Equal?(x=w639, y=w640) -> (x != y?=w641:bool)
                  }
                  frame True {
                    n231 = Not Equal?(x=w642, y=w648) -> (x != y?=w645:bool)
                    n232 = Build Path(base path=w642, name or relative path="private" ("element")) -> (appended path=w647:path)
                    n233 = Not Equal?(x=w647, y=w648) -> (x != y?=w644:bool)
                    n234 = And(x=w645, y=w644) -> (x .and. y?=w646:bool)
                  }
                }
                n235 = Search 1D Array(1D array=w629, element=w600) -> (index of element=w630:i32)  [unwired: 1 out]
                n236 = Array Size(array=w618) -> (size(s)=w617:i32)
                n237 = Greater Than 0?(x=w626) -> (x > 0?=w614:bool)
                n238 = Greater Than 0?(x=w617) -> (x > 0?=w616:bool)
                n239 = Less Than 0?(x=w630) -> (x < 0?=w590:bool)
                n240 = Strip Path(path=w600) -> (stripped path=w597:path, name=w598:string)
                n241 = Or(x=w614, y=w616) -> (x .or. y?=w615:bool)
                n242 = Not Equal?(x=w598, y="private" ("element")) -> (x != y?=w601:bool)
                n243 = Less Than 0?(x=w605) -> (x < 0?=w604:bool)
                n244 = Compound Arithmetic op=AND(w596, invert w623, w615) -> (w592:bool)
                n245 = Select(t=w600, s=w601, f=w597) -> (s? t:f=w599:path)
                n246 = Compound Arithmetic op=AND(w604, w607, w596) -> (w613:bool)
                n247 = And(x=w592, y=w590) -> (x .and. y?=w591:bool)
                n248 = case shown="True" w592 {
                  tunnel: w595 -> [w631 w634]
                  tunnel: [w631 w633] -> w593
                  tunnel: w594 -> [_ w632]
                  frame False {
                  }
                  frame True {
                    n249 = Build Array (concatenate)(w634, w632) -> (w633:path[])
                  }
                }
                n250 = case shown="True" w613 {
                  tunnel: w612 -> [w635 w638]
                  tunnel: w600 -> [_ w637]
                  tunnel: [w635 w636] -> w611
                  frame False {
                  }
                  frame True {
                    n251 = Build Array (concatenate)(w638, w637) -> (w636:path[])
                  }
                }
                n252 = case shown="True" w591 {
                  tunnel: w629 -> [w653 w656]
                  tunnel: [w653 w655] -> w628
                  tunnel: w599 -> [_ w654]
                  frame False {
                  }
                  frame True {
                    n253 = Build Array (concatenate)(w656, w654) -> (w655:path[])
                  }
                }
              }
              n254 = Bundle(cluster=w577, "Method/VI"=w579, "SubVIs/Ctls"=w580) -> (w578:T8)  [unwired: 4 in]
            }
            n255 = Bundle By Name(cluster=w571, "CreateClassVIsCalled"=w567, "dependencyClassPath"=w568, "depMethodVIs"=w565) -> (w576:T9)
          }
          frame "GetObjectAttributsDepenencies" {
            n256 = Unbundle By Name(w668) -> ("dirClass"=w659:bool, "classPath"=w657:path, "className"=w671:string)
            n257 = Concatenate Strings(w671, "ObjectAttributes.ctl" ("string")) -> (w670:string)
            n258 = case shown="True" w659 {
              tunnel: w657 -> [w673 w675]
              tunnel: [w673 w676] -> w658
              frame False {
              }
              frame True {
                n259 = Build Path(base path=w675, name or relative path="private" ("element")) -> (appended path=w676:path)
              }
            }
            n260 = Build Path(base path=w658, name or relative path=w670) -> (appended path=w663:path)
            n261 = call <resource>:"ReversedEngineering GetClassAttrubutes.vi"("Path(CtrlRenumf used if Path is empty)"=w663, "error in (no error)"=w661) -> ("attributeInfo"=w660:T2[], "error out"=w662:errorcluster)  [unwired: 1 in, 15 out]
            n262 = call <resource>:"ReversedEngineering GetObjectRefsFromPanel.vi"("Path"=w663, "error in (no error)"=w662) -> ("objectRefsFound"=w665:path[], "array"=w664:bool[], "error out"=w666:errorcluster)  [unwired: 15 out]
            n263 = Bundle By Name(cluster=w668, "objectRefsInAttrib"=w665, "objectRefInAttribIsAnArray"=w664, "objectAttribInfo"=w660) -> (w669:T9)
          }
          frame "GetClassAttributsDepenencies" {
            n264 = Unbundle By Name(w689) -> ("dirClass"=w678:bool, "classPath"=w679:path, "className"=w696:string)
            n265 = Concatenate Strings(w696, "ClassAttributes.ctl" ("string")) -> (w695:string)
            n266 = case shown="True" w678 {
              tunnel: w679 -> [w697 w699]
              tunnel: [w697 w700] -> w677
              frame False {
              }
              frame True {
                n267 = Build Path(base path=w699, name or relative path="private" ("element")) -> (appended path=w700:path)
              }
            }
            n268 = Unbundle By Name(w689) -> ("objectRefsInAttrib"=w691:path[], "objectRefInAttribIsAnArray"=w686:bool[])
            n269 = Build Path(base path=w677, name or relative path=w695) -> (appended path=w683:path)
            n270 = call <resource>:"ReversedEngineering GetClassAttrubutes.vi"("Path(CtrlRenumf used if Path is empty)"=w683, "error in (no error)"=w681) -> ("attributeInfo"=w680:T2[], "error out"=w682:errorcluster)  [unwired: 1 in, 15 out]
            n271 = call <resource>:"ReversedEngineering GetObjectRefsFromPanel.vi"("Path"=w683, "error in (no error)"=w682) -> ("objectRefsFound"=w688:path[], "array"=w685:bool[], "error out"=w694:errorcluster)  [unwired: 15 out]
            n272 = Build Array (concatenate)(w691, w688) -> (w692:path[])
            n273 = Build Array (concatenate)(w686, w685) -> (w687:bool[])
            n274 = Bundle By Name(cluster=w689, "objectRefsInAttrib"=w692, "objectRefInAttribIsAnArray"=w687, "classAttribInfo"=w680) -> (w690:T9)
          }
          frame "CloseRefs" {
            n275 = Unbundle By Name(w702) -> ("depClassDescRefs"=w704:refnum<vi>[])
            n276 = for {
              tunnel: w704 -> [w708] mode=indexing
              shift-right: [w706] -> w701
              shift-left: w703 -> [w707]
              n277 = call <resource>:"ReversedEngineering ViCachMemory.vi"("ViRef"=w708, "error in (no error)"=w707) -> ("error out"=w706:errorcluster)  [unwired: 2 in, 15 out]
            }
          }
          frame "Evaluate" {
            w716 = path[] []
            # "-2 =>  2.."
            n278 = Unbundle By Name(w710) -> ("CreateClassVIsCalled"=w714:path[], "dependencyClassPath"=w718:path[], "depClassPaths"=w721:path[], "noOfObjects1"=w722:i32[], "objectAttribInfo"=w713:T2[], "classAttribInfo"=w712:T2[])
            n279 = Build Array (concatenate)(w713, w712) -> (w711:T2[])
            n280 = Unbundle By Name(w710) -> ("IsDependencyClassPathsAByValueClass"=w709:bool[])
            n281 = for {
              tunnel: w718 -> [w735] mode=indexing
              shift-right: [w752] -> w723
              shift-left: w716 -> [w753]
              shift-right: [w751] -> w724
              shift-left: w716 -> [w750]
              tunnel: w721 -> [w749]
              tunnel: w722 -> [w748]
              shift-right: [w745] -> w720
              shift-left: i32[] [] -> [w746]
              shift-right: [w742] -> w715
              shift-left: i32[] [] -> [w743]
              tunnel: w714 -> [w739]
              tunnel: w711 -> [w734]
              tunnel: w709 -> [w730]
              i -> [w729]
              # "Use minus to indicate x.."
              n282 = Search 1D Array(1D array=w749, element=w735) -> (index of element=w747:i32)  [unwired: 1 out]
              n283 = disable-structure shown="Disabled" {
                disable-tunnel: w735 -> [w754 _]
                frame Disabled {
                  n284 = call <resource>:"ReversedEngineering GetClassObjectRefPath.vi"("llbClassPath"=w754) -> ()  [unwired: 17 in, 2 out]
                }
                frame Enabled {
                }
              }
              n285 = Index Array(array=w748, index=w747) -> (element=w736:i32)
              n286 = Greater Than 0?(x=w736) -> ()  [unwired: 1 out]
              n287 = Search 1D Array(1D array=w739, element=w735) -> (index of element=w738:i32)  [unwired: 1 out]
              n288 = Greater Or Equal To 0?(x=w738) -> (x >= 0?=w733:bool)
              n289 = call <resource>:"ReversedEngineering CountNoOfObjectAggregations.vi"("Path"=w735, "appended array"=w734) -> ("minAggregations"=w740:i32, "anyFound"=w744:bool, "noFoundLImit"=w741:bool)  [unwired: 1 in, 14 out]
              n290 = Index Array(array=w730, index=w729) -> (element=w728:bool)
              n291 = Or(x=w733, y=w728) -> (x .or. y?=w731:bool)
              n292 = case shown="True" w741 {
                tunnel: w740 -> [w755 w757]
                tunnel: [w755 w756] -> w732
                frame False {
                }
                frame True {
                  n293 = Negate(x=w757) -> (-x=w756:i32)
                }
              }
              n294 = And(x=w731, y=w744) -> (x .and. y?=w737:bool)
              n295 = case shown="False" w737 {
                tunnel: w753 -> [w766 w782]
                tunnel: [w766 w781] -> w752
                tunnel: w735 -> [w763 w780]
                tunnel: [w764 w779] -> w751
                tunnel: w750 -> [w765 w779]
                tunnel: w746 -> [w762 w778]
                tunnel: w732 -> [_ w777]
                tunnel: [w762 w776] -> w745
                tunnel: w744 -> [w761 _]
                tunnel: w732 -> [w760 _]
                tunnel: w743 -> [w759 w775]
                tunnel: [w758 w775] -> w742
                frame False {
                  n296 = case shown="False" w761 {
                    tunnel: w765 -> [w768 w774]
                    tunnel: [w768 w773] -> w764
                    tunnel: w763 -> [_ w772]
                    tunnel: w760 -> [_ w771]
                    tunnel: w759 -> [w767 w770]
                    tunnel: [w767 w769] -> w758
                    frame False {
                      # "Dependency"
                    }
                    frame True {
                      # "Aggregation"
                      n297 = Build Array (concatenate)(w774, w772) -> (w773:path[])
                      n298 = Build Array (concatenate)(w770, w771) -> (w769:i32[])
                    }
                  }
                }
                frame True {
                  # "Composite\nAggregation"
                  n299 = Build Array (concatenate)(w782, w780) -> (w781:path[])
                  n300 = Build Array (concatenate)(w778, w777) -> (w776:i32[])
                }
              }
            }
            n301 = Bundle By Name(cluster=w710, "compositeAggregationClassPath"=w723, "noOfCompositeObjects"=w720, "aggregationClassPath"=w724, "noOfAggObjects"=w715, "dependencyClassPath"=w718) -> (w725:T9)
          }
          frame "RemoveInheritDependency" {
            n302 = Unbundle By Name(w789) -> ("baseClasses"=w787:path[], "dependencyClassPath"=w788:path[], "compositeAggregationClassPath"=w784:path[], "aggregationClassPath"=w783:path[])
            n303 = for {
              tunnel: w788 -> [w799] mode=indexing
              tunnel: w787 -> [w802]
              shift-right: [w800] -> w785
              shift-left: path[] [] -> [w801]
              tunnel: w784 -> [w798]
              tunnel: w783 -> [w797]
              n304 = Search 1D Array(1D array=w802, element=w799) -> (index of element=w796:i32)  [unwired: 1 out]
              n305 = Search 1D Array(1D array=w798, element=w799) -> (index of element=w794:i32)  [unwired: 1 out]
              n306 = Search 1D Array(1D array=w797, element=w799) -> (index of element=w793:i32)  [unwired: 1 out]
              n307 = Compound Arithmetic op=ADD(w796, w794, w793) -> (w795:i32)
              n308 = case shown="-3" w795 {
                tunnel: w801 -> [w803 w806]
                tunnel: [w803 w805] -> w800
                tunnel: w799 -> [_ w804]
                frame Default {
                }
                frame -3 {
                  n309 = Build Array (concatenate)(w806, w804) -> (w805:path[])
                }
              }
            }
            n310 = Bundle By Name(cluster=w789, "dependencyClassPath"=w785) -> (w790:T9)
          }
          frame "CreateTypeDefs?" {
            n311 = Unbundle By Name(w808) -> ("objectAttribInfo"=w818:T2[], "classAttribInfo"=w817:T2[])
            n312 = Build Array (concatenate)(w818, w817) -> (w816:T2[])
            n313 = for {
              tunnel: w816 -> [w863] mode=indexing
              shift-right: [w864] -> w812
              shift-left: T1[] [] ("TypeDefs") -> [w860]
              n314 = Unbundle By Name(w863) -> ("type"=w862:T3, "typeName"=w849:string, "typePath"=w852:path)
              n315 = call <resource>:"ReversedEngineering GetClassAttrubutes.vi"("Path(CtrlRenumf used if Path is empty)"=w852) -> ("LibraryName"=w851:string, "attributeInfo"=w858:T2[], "error out"=w857:errorcluster)  [unwired: 2 in, 14 out]
              n316 = Equal?(x=w862, y=CommonVIs_AttributeDataType."TypeDef") -> (x = y?=w856:bool)
              n317 = case shown="\"False\", Default" w851 {
                selector: w851 -> [w868 _]
                tunnel: [w865 w869] -> w850
                tunnel: w849 -> [w866 w869]
                frame "False", Default {
                  n318 = Format Into String(format string="%s : %s", w868, w866) -> (resulting string=w865:string)  [unwired: 2 in, 1 out]
                }
                frame "" {
                }
              }
              n319 = Unbundle By Name(w857) -> ("status"=w855:bool)
              n320 = Compound Arithmetic op=AND(w856, invert w855) -> (w854:bool)
              n321 = Index Array(array=w860) -> (element=w859:T1)  [unwired: 1 in]
              n322 = Bundle By Name(cluster=w859, "TypeDefName"=w850, "TypeDefPath"=w852, "TypeDefAttribInfo"=w858) -> (w853:T1)
              n323 = case shown="True" w854 {
                tunnel: w860 -> [w870 w873]
                tunnel: [w870 w872] -> w864
                tunnel: w853 -> [_ w871]
                frame False {
                }
                frame True {
                  n324 = Build Array (concatenate)(w873, w871) -> (w872:T1[])
                }
              }
            }
            n325 = for {
              tunnel: w812 -> [w823] mode=indexing
              shift-right: [w820] -> w810
              shift-left: T1[] [] ("TypeDefs") -> [w821]
              n326 = Unbundle By Name(w823) -> ("TypeDefAttribInfo"=w822:T2[])
              n327 = for {
                tunnel: w822 -> [w838] mode=indexing
                shift-right: [w839] -> w820
                shift-left: w821 -> [w835]
                n328 = Unbundle By Name(w838) -> ("type"=w837:T3, "typeName"=w825:string, "typePath"=w827:path)
                n329 = Equal?(x=w837, y=CommonVIs_AttributeDataType."TypeDef") -> (x = y?=w831:bool)
                n330 = call <resource>:"ReversedEngineering GetClassAttrubutes.vi"("Path(CtrlRenumf used if Path is empty)"=w827) -> ("LibraryName"=w826:string, "attributeInfo"=w833:T2[], "error out"=w832:errorcluster)  [unwired: 2 in, 14 out]
                n331 = case shown="\"False\", Default" w826 {
                  selector: w826 -> [w843 _]
                  tunnel: [w840 w844] -> w824
                  tunnel: w825 -> [w841 w844]
                  frame "False", Default {
                    n332 = Format Into String(format string="%s : %s", w843, w841) -> (resulting string=w840:string)  [unwired: 2 in, 1 out]
                  }
                  frame "" {
                  }
                }
                n333 = Unbundle By Name(w832) -> ("status"=w830:bool)
                n334 = Compound Arithmetic op=AND(w831, invert w830) -> (w829:bool)
                n335 = Index Array(array=w835) -> (element=w834:T1)  [unwired: 1 in]
                n336 = Bundle By Name(cluster=w834, "TypeDefName"=w824, "TypeDefPath"=w827, "TypeDefAttribInfo"=w833) -> (w828:T1)
                n337 = case shown="True" w829 {
                  tunnel: w835 -> [w845 w848]
                  tunnel: [w845 w847] -> w839
                  tunnel: w828 -> [_ w846]
                  frame False {
                  }
                  frame True {
                    n338 = Build Array (concatenate)(w848, w846) -> (w847:T1[])
                  }
                }
              }
            }
            n339 = Unbundle By Name(w808) -> ("TypeDefs"=w807:T1[])
            n340 = Build Array (concatenate)(w807, w812, w810) -> (w809:T1[])
            n341 = Bundle By Name(cluster=w808, "TypeDefs"=w809) -> (w815:T9)
          }
          frame "AddReferencedTypeDefs" {
            n342 = Unbundle By Name(w881) -> ("TypeDefs"=w874:T1[], "depMethodVIs"=w876:T8[])
            n343 = for {
              tunnel: w874 -> [w883] mode=indexing
              tunnel: [w882] -> w875 mode=indexing
              n344 = Unbundle By Name(w883) -> ("TypeDefPath"=w882:path)
            }
            n345 = for {
              shift-right: [w885] -> w878
              shift-left: w874 -> [w884]
              tunnel: w876 -> [w891] mode=indexing
              shift-right: [w888] -> _
              shift-left: w875 -> [w889]
              n346 = Unbundle By Name(w891) -> ("SubVIs/Ctls"=w890:path[], "SubVIClassOwner"=w887:string[], "ClassMethodName"=w886:string[])
              n347 = for {
                tunnel: w890 -> [w894] mode=indexing
                shift-right: [w899] -> w885
                shift-left: w884 -> [w900]
                shift-right: [w898] -> w888
                shift-left: w889 -> [w901]
                tunnel: w887 -> [w897] mode=indexing
                tunnel: w886 -> [w896] mode=indexing
                n348 = Strip Path(path=w894) -> (stripped path=w893:path)  [unwired: 1 out]
                n349 = call <vilib>:"Get File Extension.vi"("file"=w893) -> ("lowercase file extension"=w892:string)  [unwired: 1 in, 9 out]
                n350 = call <vilib>:"Get File Extension.vi"("file"=w894) -> ("filename without extension"=w895:string, "lowercase file extension"=w903:string, "dup file"=w902:path)  [unwired: 1 in, 7 out]
                n351 = case shown="\"ctl\", \"ctt\"" w903 {
                  tunnel: w902 -> [_ w908]
                  tunnel: w901 -> [w904 w911]
                  tunnel: w900 -> [w905 w912]
                  tunnel: [w905 w910] -> w899
                  tunnel: [w904 w909] -> w898
                  tunnel: w897 -> [_ _]
                  tunnel: w896 -> [_ _]
                  tunnel: w895 -> [_ w907]
                  tunnel: w892 -> [_ w906]
                  frame "False", Default {
                  }
                  frame "ctl", "ctt" {
                    n352 = case shown="\"lvclass\"" w906 {
                      tunnel: w912 -> [w914 w920]
                      tunnel: w911 -> [w913 w919]
                      tunnel: [w914 w918] -> w910
                      tunnel: [w913 w917] -> w909
                      tunnel: w908 -> [_ w916]
                      tunnel: w907 -> [_ w915]
                      frame "lvclass" {
                      }
                      frame Default {
                        n353 = Search 1D Array(1D array=w919, element=w916) -> (index of element=w921:i32)  [unwired: 1 out]
                        n354 = case shown="-1" w921 {
                          tunnel: w920 -> [w923 w938]
                          tunnel: w919 -> [w922 w936]
                          tunnel: [w923 w937] -> w918
                          tunnel: [w922 w935] -> w917
                          tunnel: w916 -> [_ w930]
                          tunnel: w915 -> [_ w932]
                          frame 0, Default {
                          }
                          frame -1 {
                            n355 = call <resource>:"ReversedEngineering GetClassAttrubutes.vi"("Path(CtrlRenumf used if Path is empty)"=w930) -> ("LibraryName"=w929:string, "attributeInfo"=w928:T2[], "error out"=w927:errorcluster)  [unwired: 2 in, 14 out]
                            n356 = case shown="\"False\", Default" w929 {
                              selector: w929 -> [w950 _]
                              tunnel: [w947 w951] -> w931
                              tunnel: w932 -> [w948 w951]
                              frame "False", Default {
                                n357 = Format Into String(format string="%s : %s", w950, w948) -> (resulting string=w947:string)  [unwired: 2 in, 1 out]
                              }
                              frame "" {
                              }
                            }
                            n358 = Unbundle(w927) -> ("status"=w925:bool)  [unwired: 2 out]
                            n359 = Empty Array?(array=w928) -> (empty?=w926:bool)
                            n360 = Or(x=w926, y=w925) -> (x .or. y?=w924:bool)
                            n361 = Bundle(cluster=T1 {"TypeDefName"="", "TypeDefPath"=path "", "TypeDefAttribInfo"=[]} ("TypeDef"), "TypeDefName"=w931, "TypeDefPath"=w930, "TypeDefAttribInfo"=w928) -> (w933:T1)
                            n362 = case shown="False" w924 {
                              tunnel: w938 -> [w944 w946]
                              tunnel: [w943 w946] -> w937
                              tunnel: w936 -> [w942 w945]
                              tunnel: [w941 w945] -> w935
                              tunnel: w933 -> [w940 _]
                              tunnel: w930 -> [w939 _]
                              frame False {
                                n363 = Build Array (concatenate)(w944, w940) -> (w943:T1[])
                                n364 = Build Array (concatenate)(w942, w939) -> (w941:path[])
                              }
                              frame True {
                              }
                            }
                          }
                        }
                      }
                    }
                  }
                }
              }
            }
            n365 = Bundle By Name(cluster=w881, "TypeDefs"=w878) -> (w880:T9)
          }
          frame "UpdateTypeDefsAttribName?" {
            n366 = Unbundle By Name(w961) -> ("objectAttribInfo"=w958:T2[], "classAttribInfo"=w956:T2[], "TypeDefs"=w953:T1[])
            n367 = for {
              tunnel: w953 -> [w964] mode=indexing
              tunnel: [w962] -> w952 mode=indexing
              n368 = Unbundle By Name(w964) -> ("TypeDefAttribInfo"=w965:T2[])
              n369 = for {
                tunnel: w965 -> [w968] mode=indexing
                tunnel: [w967] -> w963 mode=indexing
                n370 = Unbundle By Name(w968) -> ("type"=w975:T3, "typeName"=w972:string)
                n371 = Equal?(x=w975, y=CommonVIs_AttributeDataType."TypeDef") -> (x = y?=w969:bool)
                n372 = String To Path(string=w972) -> (path=w970:path)
                n373 = Strip Path(path=w970) -> (name=w973:string)  [unwired: 1 out]
                n374 = Match Pattern(string=w973, regular expression="[.][cC][tT][lL]$") -> (before substring=w966:string)  [unwired: 4 out]
                n375 = case shown="True" w969 {
                  tunnel: w968 -> [w976 w979]
                  tunnel: [w976 w978] -> w967
                  tunnel: w966 -> [_ w977]
                  frame False {
                  }
                  frame True {
                    n376 = Bundle By Name(cluster=w979, "typeName"=w977) -> (w978:T2)
                  }
                }
              }
              n377 = Bundle By Name(cluster=w964, "TypeDefAttribInfo"=w963) -> (w962:T1)
            }
            n378 = for {
              tunnel: w958 -> [w996] mode=indexing
              tunnel: [w995] -> w957 mode=indexing
              n379 = Unbundle By Name(w996) -> ("type"=w1003:T3, "typeName"=w1000:string)
              n380 = Equal?(x=w1003, y=CommonVIs_AttributeDataType."TypeDef") -> (x = y?=w997:bool)
              n381 = String To Path(string=w1000) -> (path=w998:path)
              n382 = Strip Path(path=w998) -> (name=w1001:string)  [unwired: 1 out]
              n383 = Match Pattern(string=w1001, regular expression="[.][cC][tT][lL]$") -> (before substring=w994:string)  [unwired: 4 out]
              n384 = case shown="True" w997 {
                tunnel: w996 -> [w1004 w1007]
                tunnel: [w1004 w1006] -> w995
                tunnel: w994 -> [_ w1005]
                frame False {
                }
                frame True {
                  n385 = Bundle By Name(cluster=w1007, "typeName"=w1005) -> (w1006:T2)
                }
              }
            }
            n386 = for {
              tunnel: w956 -> [w982] mode=indexing
              tunnel: [w981] -> w955 mode=indexing
              n387 = Unbundle By Name(w982) -> ("type"=w989:T3, "typeName"=w986:string)
              n388 = Equal?(x=w989, y=CommonVIs_AttributeDataType."TypeDef") -> (x = y?=w983:bool)
              n389 = String To Path(string=w986) -> (path=w984:path)
              n390 = Strip Path(path=w984) -> (name=w987:string)  [unwired: 1 out]
              n391 = Match Pattern(string=w987, regular expression="[.][cC][tT][lL]$") -> (before substring=w980:string)  [unwired: 4 out]
              n392 = case shown="True" w983 {
                tunnel: w982 -> [w990 w993]
                tunnel: [w990 w992] -> w981
                tunnel: w980 -> [_ w991]
                frame False {
                }
                frame True {
                  n393 = Bundle By Name(cluster=w993, "typeName"=w991) -> (w992:T2)
                }
              }
            }
            n394 = Bundle By Name(cluster=w961, "objectAttribInfo"=w957, "classAttribInfo"=w955, "TypeDefs"=w952) -> (w960:T9)
          }
          frame "SortMethodToClassDependencies" {
            w1010 = cluster{path[]}[] []
            n395 = Unbundle By Name(w1017) -> ("depMethodVIs"=w1014:T8[])
            n396 = for {
              shift-right: [w1039] -> w1016
              shift-left: path[] [] -> [w1041]
              shift-right: [w1038] -> w1012
              shift-left: w1010 -> [w1035]
              tunnel: w1014 -> [w1042] mode=indexing
              shift-right: [w1036] -> w1011
              shift-left: w1010 -> [w1034]
              shift-right: [w1032] -> w1008
              shift-left: cluster{T7[]}[] [] -> [w1030]
              n397 = Unbundle(w1042) -> ("Method/VI"=w1037:path, "SubVIs/Ctls"=w1040:path[], "SubVIClassOwnerPath"=w1033:path[], "DepType"=w1031:T7[])  [unwired: 2 out]
              n398 = for {
                shift-right: [w1055] -> w1039
                shift-left: w1041 -> [w1054]
                tunnel: w1040 -> [w1047] mode=indexing
                shift-right: [w1051] -> w1038
                shift-left: w1035 -> [w1052]
                tunnel: w1037 -> [w1050]
                shift-right: [w1049] -> w1036
                shift-left: w1034 -> [w1048]
                tunnel: w1033 -> [w1046] mode=indexing
                shift-right: [w1044] -> w1032
                shift-left: w1030 -> [w1045]
                tunnel: w1031 -> [w1043] mode=indexing
                # "ConvertTo\nClassPath"
                n399 = Search 1D Array(1D array=w1054, element=w1046) -> (index of element=w1053:i32)  [unwired: 1 out]
                n400 = case shown="Default" w1053 {
                  selector: w1053 -> [w1056 _]
                  tunnel: [w1078 w1094] -> w1055
                  tunnel: w1046 -> [_ w1096]
                  tunnel: w1054 -> [w1078 w1095]
                  tunnel: w1052 -> [w1073 w1091]
                  tunnel: [w1072 w1090] -> w1051
                  tunnel: w1050 -> [w1075 w1089]
                  tunnel: w1048 -> [w1065 w1086]
                  tunnel: [w1066 w1087] -> w1049
                  tunnel: w1047 -> [w1064 w1088]
                  tunnel: w1045 -> [w1062 w1081]
                  tunnel: [w1061 w1080] -> w1044
                  tunnel: w1043 -> [w1063 w1079]
                  frame Default {
                    n401 = Index Array(array=w1073, index=w1056) -> (element=w1077:cluster{path[]})
                    n402 = Index Array(array=w1065, index=w1056) -> (element=w1067:cluster{path[]})
                    n403 = Index Array(array=w1062, index=w1056) -> (element=w1060:cluster{T7[]})
                    n404 = Unbundle(w1077) -> (w1076:path[])
                    n405 = Unbundle(w1067) -> (w1068:path[])
                    n406 = Unbundle(w1060) -> (w1059:T7[])
                    n407 = Build Array (concatenate)(w1076, w1075) -> (w1074:path[])
                    n408 = Build Array (concatenate)(w1068, w1064) -> (w1069:path[])
                    n409 = Build Array (concatenate)(w1059, w1063) -> (w1058:T7[])
                    n410 = Bundle(w1074) -> (w1071:cluster{path[]})  [unwired: 1 in]
                    n411 = Bundle(w1069) -> (w1070:cluster{path[]})  [unwired: 1 in]
                    n412 = Bundle(w1058) -> (w1057:cluster{T7[]})  [unwired: 1 in]
                    n413 = Replace Array Subset(array=w1073, new element=w1071, index=w1056) -> (w1072:cluster{path[]}[])
                    n414 = Replace Array Subset(array=w1065, new element=w1070, index=w1056) -> (w1066:cluster{path[]}[])
                    n415 = Replace Array Subset(array=w1062, new element=w1057, index=w1056) -> (w1061:cluster{T7[]}[])
                  }
                  frame -1 {
                    n416 = Build Array(w1089) -> (w1092:path[])
                    n417 = Build Array(w1088) -> (w1085:path[])
                    n418 = Bundle(w1092) -> (w1093:cluster{path[]})  [unwired: 1 in]
                    n419 = Bundle(w1085) -> (w1084:cluster{path[]})  [unwired: 1 in]
                    n420 = Build Array(w1079) -> (w1082:T7[])
                    n421 = Build Array (concatenate)(w1095, w1096) -> (w1094:path[])
                    n422 = Build Array (concatenate)(w1091, w1093) -> (w1090:cluster{path[]}[])
                    n423 = Build Array (concatenate)(w1086, w1084) -> (w1087:cluster{path[]}[])
                    n424 = Bundle(w1082) -> (w1083:cluster{T7[]})  [unwired: 1 in]
                    n425 = Build Array (concatenate)(w1081, w1083) -> (w1080:cluster{T7[]}[])
                  }
                }
              }
            }
            n426 = for {
              tunnel: w1016 -> [w1028] mode=indexing
              tunnel: [w1026] -> w1015 mode=indexing
              tunnel: w1012 -> [w1025] mode=indexing
              tunnel: w1011 -> [w1024] mode=indexing
              tunnel: w1008 -> [w1022] mode=indexing
              n427 = Unbundle(w1025) -> (w1027:path[])
              n428 = Unbundle(w1024) -> (w1023:path[])
              n429 = Unbundle(w1022) -> (w1021:T7[])
              n430 = Bundle(cluster=T6 {"DepClassPath"=path "", "ThisVIs/Ctls"=[], "Dependent_VIs/Ctls"=[], "ViDependecyType"=[]} ("DepClass"), "DepClassPath"=w1028, "ThisVIs/Ctls"=w1027, "Dependent_VIs/Ctls"=w1023, "ViDependecyType"=w1021) -> (w1026:T6)
            }
            n431 = Bundle By Name(cluster=w1017, "DependencyDetails"=w1015) -> (w1019:T9)
          }
          frame "Error", Default {
          }
        }
        n432 = call <resource>:"UMLEditor ControlBusyDialog.vi"("error in (no error)"=w49, "Action(SendStatusMessage)"=w48) -> ("error out"=w45:errorcluster)  [unwired: 2 in, 15 out]
        n433 = Equal?(x=w58, y="Exit") -> (x = y?=w56:bool)
        n434 = Or(x=w56, y=w45) -> (x .or. y?=w55:bool)
      }
    }
    frame Error {
    }
  }
  n435 = Unbundle By Name(w29) -> ("TypeDefs"=→"TypeDefs":T1[], "inherits"=w26:bool, "baseClasses"=w25:path[], "compositeAggregationClassPath"=w24:path[], "noOfCompositeObjects"=w23:i32[], "aggregationClassPath"=w22:path[], "noOfAggObjects"=w21:i32[], "dependencyClassPath"=w20:path[], "methodNames"=w19:string[], "methodPuplic"=w18:T4[], "objectAttribInfo"=w17:T2[], "classAttribInfo"=w16:T2[], "ClassDesc"=w9:string, "DependencyDetails"=w6:T6[], "Interface"=w2:bool, "ParentInterfaces"=w1:path[], "createRef"=w8:refnum<vi>, "errMsg"=w12:string)
  n436 = case shown="Error" w15 {
    selector: w15 -> [w1101 w1109]
    tunnel: [w1101 w1108] -> w14
    tunnel: w13 -> [_ w1105]
    tunnel: w12 -> [_ w1103]
    frame No Error {
    }
    frame Error {
      n437 = Unbundle By Name(w1109) -> ("code"=w1102:i32, "source"=w1104:string)
      n438 = Format Into String(format string="<ERR>\nCase:%s\nError:[%d]%s\nSource:%s", w1105, w1102, w1103, w1104) -> (resulting string=w1106:string)  [unwired: 2 in, 1 out]
      n439 = Bundle By Name(cluster=w1109, "source"=w1106) -> (w1108:errorcluster)
    }
  }
  "error out" <- w14
  n440 = call <resource>:"ReversedEngineering ViCachMemory.vi"("ViRef"=w8) -> ()  [unwired: 3 in, 16 out]
  n441 = local read "classInfo"() -> (w28:T5)
  n442 = Bundle By Name(cluster=w28, "classPath"="Class/Create Path", "inherits"=w26, "baseClasses"=w25, "compAggClasses"=w24, "noOfCompObj"=w23, "aggClasses"=w22, "noOfAgg"=w21, "depClasses"=w20, "methods"=w19, "methodPuplic"=w18, "objectAttrib"=w17, "classAttrib"=w16, "ClassDesc"=w9, "DependencyDetails"=w6, "Interface"=w2, "ParentInterfaces"=w1) -> (→"classInfo":T5)
